vi "信号光谱9 - BN_5.10.vi"() -> ()   [LabVIEW 2018]
uses:
  <vilib>/Utility/NIReport.llb/Report Type.ctl
  <vilib>/Utility/file.llb/Write Delimited Spreadsheet (DBL).vi
  <vilib>/Instr/_visa.llb/VISA Configure Serial Port (Instr).vi
  <vilib>/addons/_office/excel.llb/Excel Get Data ([str]).vi
  <vilib>/Utility/NIReport.llb/NI_report.lvclass
  <vilib>/Analysis/NI_AALBase.lvlib
  <vilib>/ptbypt/NI_PtbyPt.lvlib
  <vilib>/Utility/NIReport.llb/NI_ReportGenerationCore.lvlib
  <vilib>/addons/_office/NI_ReportGenerationToolkit.lvlib
  <vilib>/Utility/NIReport.llb/Excel/NI_Excel.lvclass
panel:
  out "error out 2":errorcluster caption="错误输出"
  out "错误输出":errorcluster
  in  "超时毫秒(25000)":i32=20000
  in  "读取的字节":i32=7
  in  "格式字符串":string
  in  "分隔符(Tab)":string=","
  in  "端口":u16=65432
  in  "地址":string="127.0.0.1"
  out "原始峰值":dbl
  out "拟合峰值":dbl
  in  "角度倍乘系数":dbl=1.5
  out "结果展示":dbl[][](array[numeric])=[[37.33100777239877, 2672.955043835526, 29.54153292599307, 222755.0, 50.0], [37.36593979472361, 2672.656498058864, 30.113284142729572, 222833.0, 50.0], [38.96986225690859, 2673.3337152325566, 33.38805102415213, 222910.0, 75.0], [37.39946104045098, 2676.4005085744548, 31.215565446104666, 222948.0, 47.0], [35.862209164247574, 2671.7826876859012, 30.355582265151796, 223028.0, 47.0]]
  out "Δw2>C":bool=TRUE
  out "Δw1>C":bool=TRUE
  out "θi":dbl
  in  "w0":dbl format="%#_13g"
  in  "C=w-w0":dbl=180.0 format="%#_13g"
  in  "上升下降沿/s":dbl format="%.2p"
  in  "延时/s":dbl format="%.2p"
  in  "占空比/%":dbl=3.0 format="%.2p"
  in  "高电平/V":dbl=4.0 format="%.2p"
  in  "频率/Hz":dbl=6000.0 format="%.3p"
  in  "低电平/V":dbl min=0.0 max=5.0 format="%.2p"
  in  "Enable":bool
  in  "上升下降沿":i32(ring)=1 items=["上升沿", "下降沿"]
  in  "输出信号波形":u16(ring) items=["Pulse"]
  out "Output":bool
  in  "VISA 信号发生器":refnum<visa-resource-name>="USB0::0x1AB1::0x0641::DG4E192200870::INSTR"
  out "Output 2":bool
  in  "Enable 2":bool
  in  "上升下降沿/s 2":dbl format="%.2p"
  in  "延时/s 2":dbl format="%.2p"
  in  "占空比/% 2":dbl=3.0 format="%.2p"
  in  "高电平/V 2":dbl=0.002 format="%.2p"
  in  "频率/Hz 2":dbl=6000.0 format="%.3p"
  in  "低电平/V 2":dbl min=0.0 max=5.0 format="%.2p"
  in  "上升下降沿 2":i32(ring)=1 items=["上升沿", "下降沿"]
  in  "输出信号波形 2":u16(ring) items=["Pulse"]
  in  "终止测量":bool
  in  "测量次数":i32=1
  out "best fit":cluster{"Y":dbl[], "Y":dbl[]}[](graph)
  in  "拟合终点":i32=850
  in  "拟合起点":i32=200
  out "angle":dbl
  out "图片地址":string
  in  "开光时间/ms":u32=50
  out "最终存储路径 2":path
  out "照明光error out":errorcluster
  in  "照明光":bool
  in  "stop bits (10: 1 bit)":u16(ring)=10 items=["1.0"=10, "1.5"=15, "2.0"=20]
  in  "parity (0:none)":enum16{"None", "Odd", "Even", "Mark", "Space"}(ring)
  in  "data bits (8)":u16=8 min=5 max=8 step=1
  in  "baud rate":u32=9600 caption="baud rate (115200)" min=9600 max=115200
  in  "照明光VISA":refnum<visa-resource-name>="COM13"
  out "正在测量":bool
  in  "滤波阈值":dbl=3000.0 format="%#_13g"
  out "范围内？":bool[](array[boolean])
  out "w":dbl
  out "xc":dbl
  out "拟合参数":dbl[](array[numeric])
  out "最终存储路径":path
  in  "停止程序":bool
  out "configure error out":errorcluster
  in  "设置参数":bool
  out "output control error  4":errorcluster
  in  "低电平持续输出":bool
  out "output control error  5":errorcluster
  out "output control error":errorcluster
  in  "开始测量":bool
  in  "channel输出口":i32(ring) items=["Channel 1", "Channel 2"]
  out "output control error":errorcluster
  out "Spectrum":cluster{"Y":dbl[], "Y":dbl[]}[](graph)
  out "波长范围":dbl[](array[numeric])
  in  "?":enum32{"IHR 550", "CCD"}(tab)
  in  "Move To\nTarget Positions":bool
  out "Current UniqueID":string="Mono4"
  in  "Mono ID":string(combo)="Mono1"
  in  "Connect":bool
  out "Initialized JY":bool=TRUE
  in  "Force\nInitialization":bool
  in  "Target Grating":string(combo)="2"
  out "Current Description":string="1" caption="Description"
  out "Grating Index":i32=1
  out "Current Grating":dbl=1200.0
  out "Units":string="nm"
  out "Current WL":dbl=897.9988
  out "Exit Mirror\nPosition":i32(ring)=2 items=["EntranceMirror", "ExitMirror", "Front", "Side"]
  out "Entrance Mirror\nPosition":i32(ring)=2 items=["EntranceMirror", "ExitMirror", "Front", "Side"]
  out "Units 2":string="mm"
  out "Front Entrance":dbl
  in  "Target WL":dbl=516.0
  in  "Exit Mirror":u16(ring)=3 caption="Target Position Exit Mirror" items=["Front"=2, "Side"=3]
  in  "Entrance Mirror":u16(ring)=2 caption="Target Position\nEntrance Mirror" items=["Front"=2, "Side"=3]
  in  "Target\nFront Entrance":dbl=2.0
  in  "Commande tab":T1(tab)
  in  "Area Number to Display":i32
  in  "Reformat":bool
  in  "GAIN":u16(ring)=2 caption="Device Name" items=["High Light", "Best Dynamic Range", "High Sensitivity"]
  in  "ADC":u16(ring) caption="Device Name" items=["20 kHz       ", " 1 MHz       ", " 1 MHz Ultra "]
  in  "Number of Areas :":u16=1 min=1 step=1
  in  "Integration time (ms) :":i16=20000
  out "Uniques ID":u16(ring) items=["CCD1", "CCD2"]
  in  "Device Name":u16(ring) items=["Synapse CCD (Lateral)", "Synapse_IGA (Axial)"]
  in  "Signal type :":enum16{"TTL Rising Edge", "TTL Falling Edge"}(ring)=enum."TTL Falling Edge"
  in  "Trigger Type :":u16(ring) items=["On Start"=1, "Per Acquisition"=2]
  in  "trigSigTypeString":string
  in  "trigEventString":string
  in  "Enable InputTriggers :":bool
  in  "Number of Cleans":i32=1
  in  "MultiAcqShutterMode":i32(ring)=3 items=["Open For All Spectra"=1, "Open for Each Spectrum"=3]
  in  "Accumulations:":u16=10 min=1 step=1
  in  "Multi Accumulation mode:":bool
  out "Y Pixels:":i32=256
  out "DataSize":i32=1024
  out "X Pixels:":i32=1024
  out "Firmware\nVersion":string="V1.20 CCD_4000"
  out "initialized ?":bool=TRUE
  in  "Continuous":bool
  in  "CCD Busy":bool
  out "indicator":string="Ready !"
  in  "initialize":bool
  in  "ShutterOpen":bool=TRUE caption="Shutter enable"
  in  "Acquire":bool
  in  "Temperature":bool
  in  "Setup":bool
  out "Acq Time(ms)":u32=3401
  in  "Save Backlight":bool
  in  "cut backlight":bool
  out "backlight":bool=TRUE
  in  "是否拟合":bool
  in  "是否保存":bool
  in  "Close":bool=TRUE
  out "JYCCDLib.IJYCCDReqd":refnum<k7>
  out "areas :":i32[][](array[numeric])=[[1], [1], [1], [1024], [256], [1], [256]]
  in  "Constante de condition\n(Voir l'aide contextuelle)":bool
  out "temp graph":dbl(graph)=-134.538067
  out "ADC Number":i32[](array[numeric])=[0, 1, 2, 3, 4]
  out "Gain Number":i32[](array[numeric])=[10, 11, 12, 13, 8, 2]
  out "trigAddress":i32
  out "Data":i32[][](graph)
  out "error out":errorcluster
  out "Gratings":dbl[](array[numeric])=[1200.0, 300.0]
  out "Backlight":i32[][](graph)
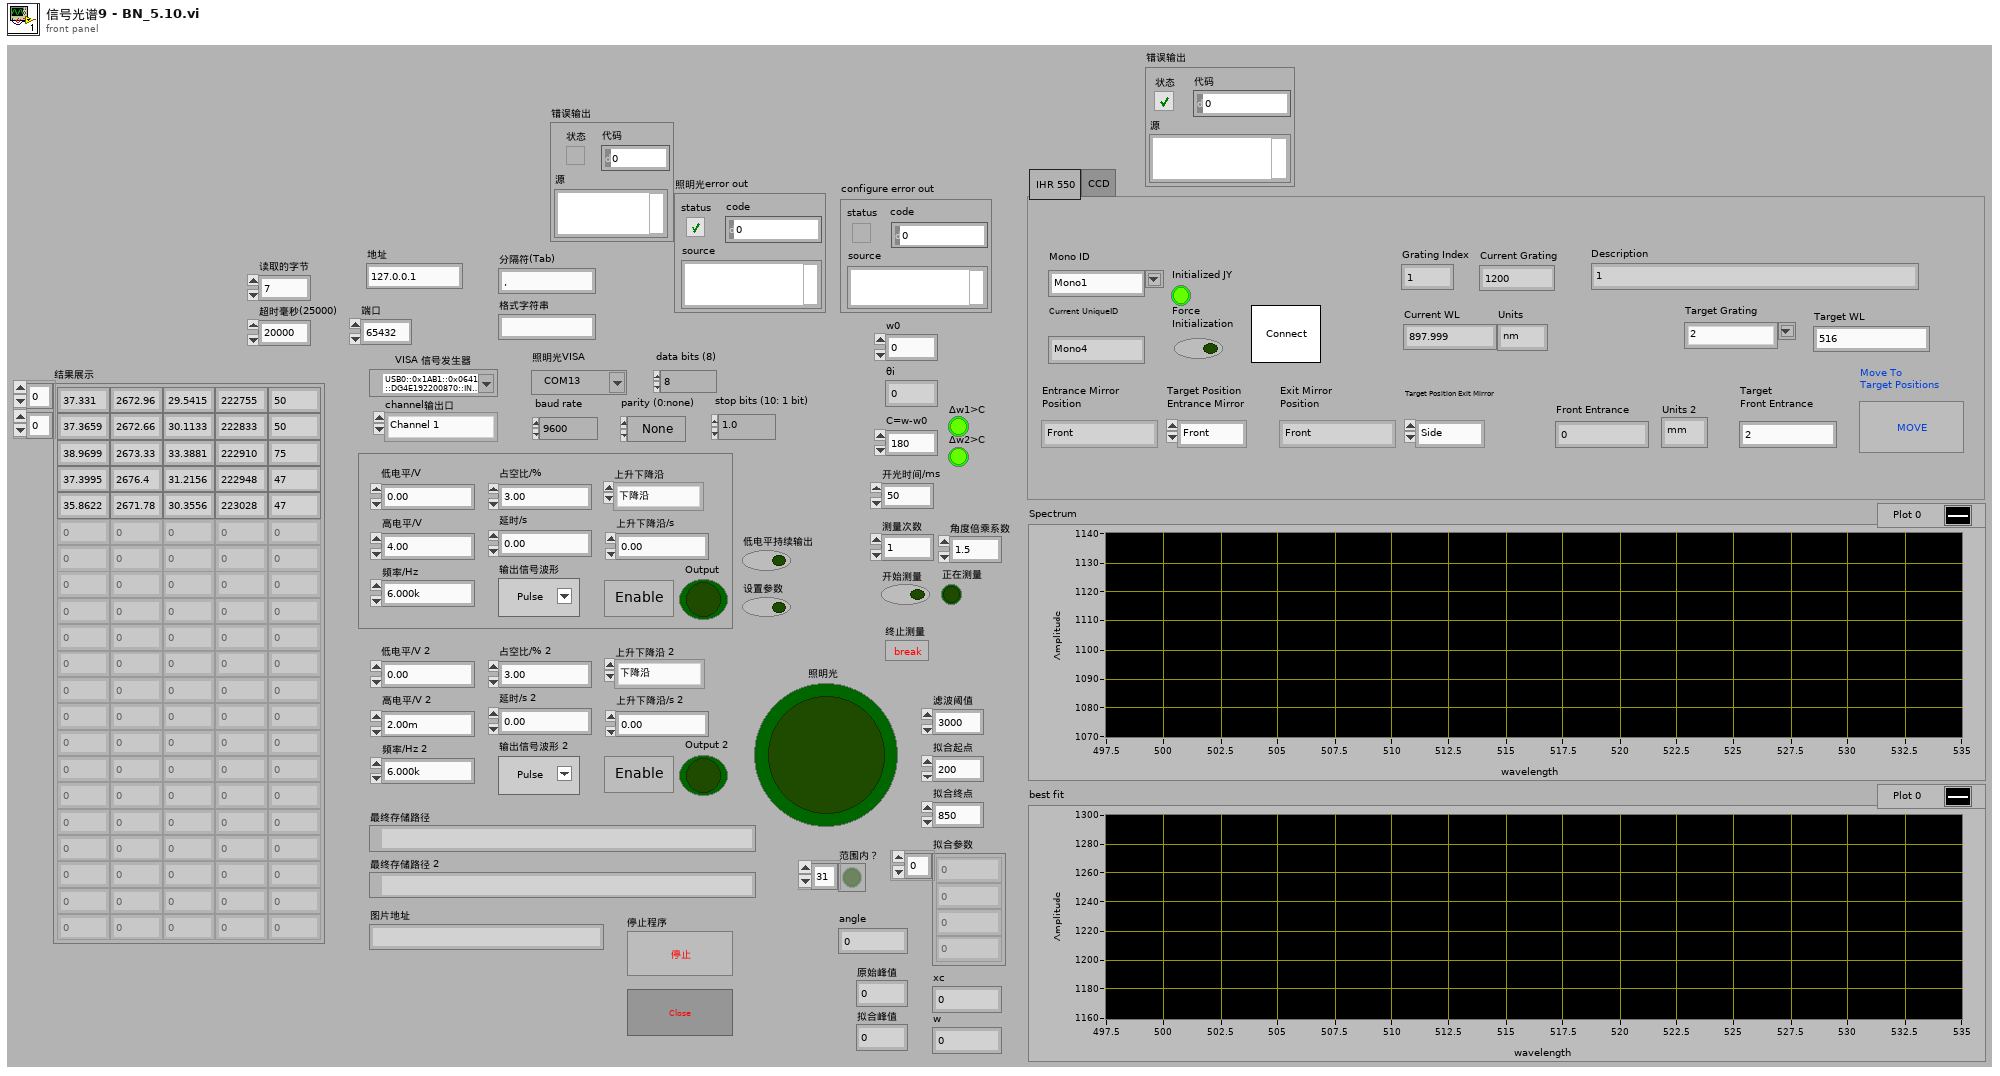
[diagram p1: front panel]
types:
  T1 = enum32{"Settings", "Trigger In", "Multi-Accu.", "Infos"}
  T2 = enum8{"Enabled", "Disabled", "Disabled and Grayed Out"}
  T3 = enum16{"maximized", "minimized", "normal", "no change"}
  T4 = typedef "NI_ReportGenerationCore.lvlib/Report Type.ctl" = enum16{"HTML", "Word", "Excel"}
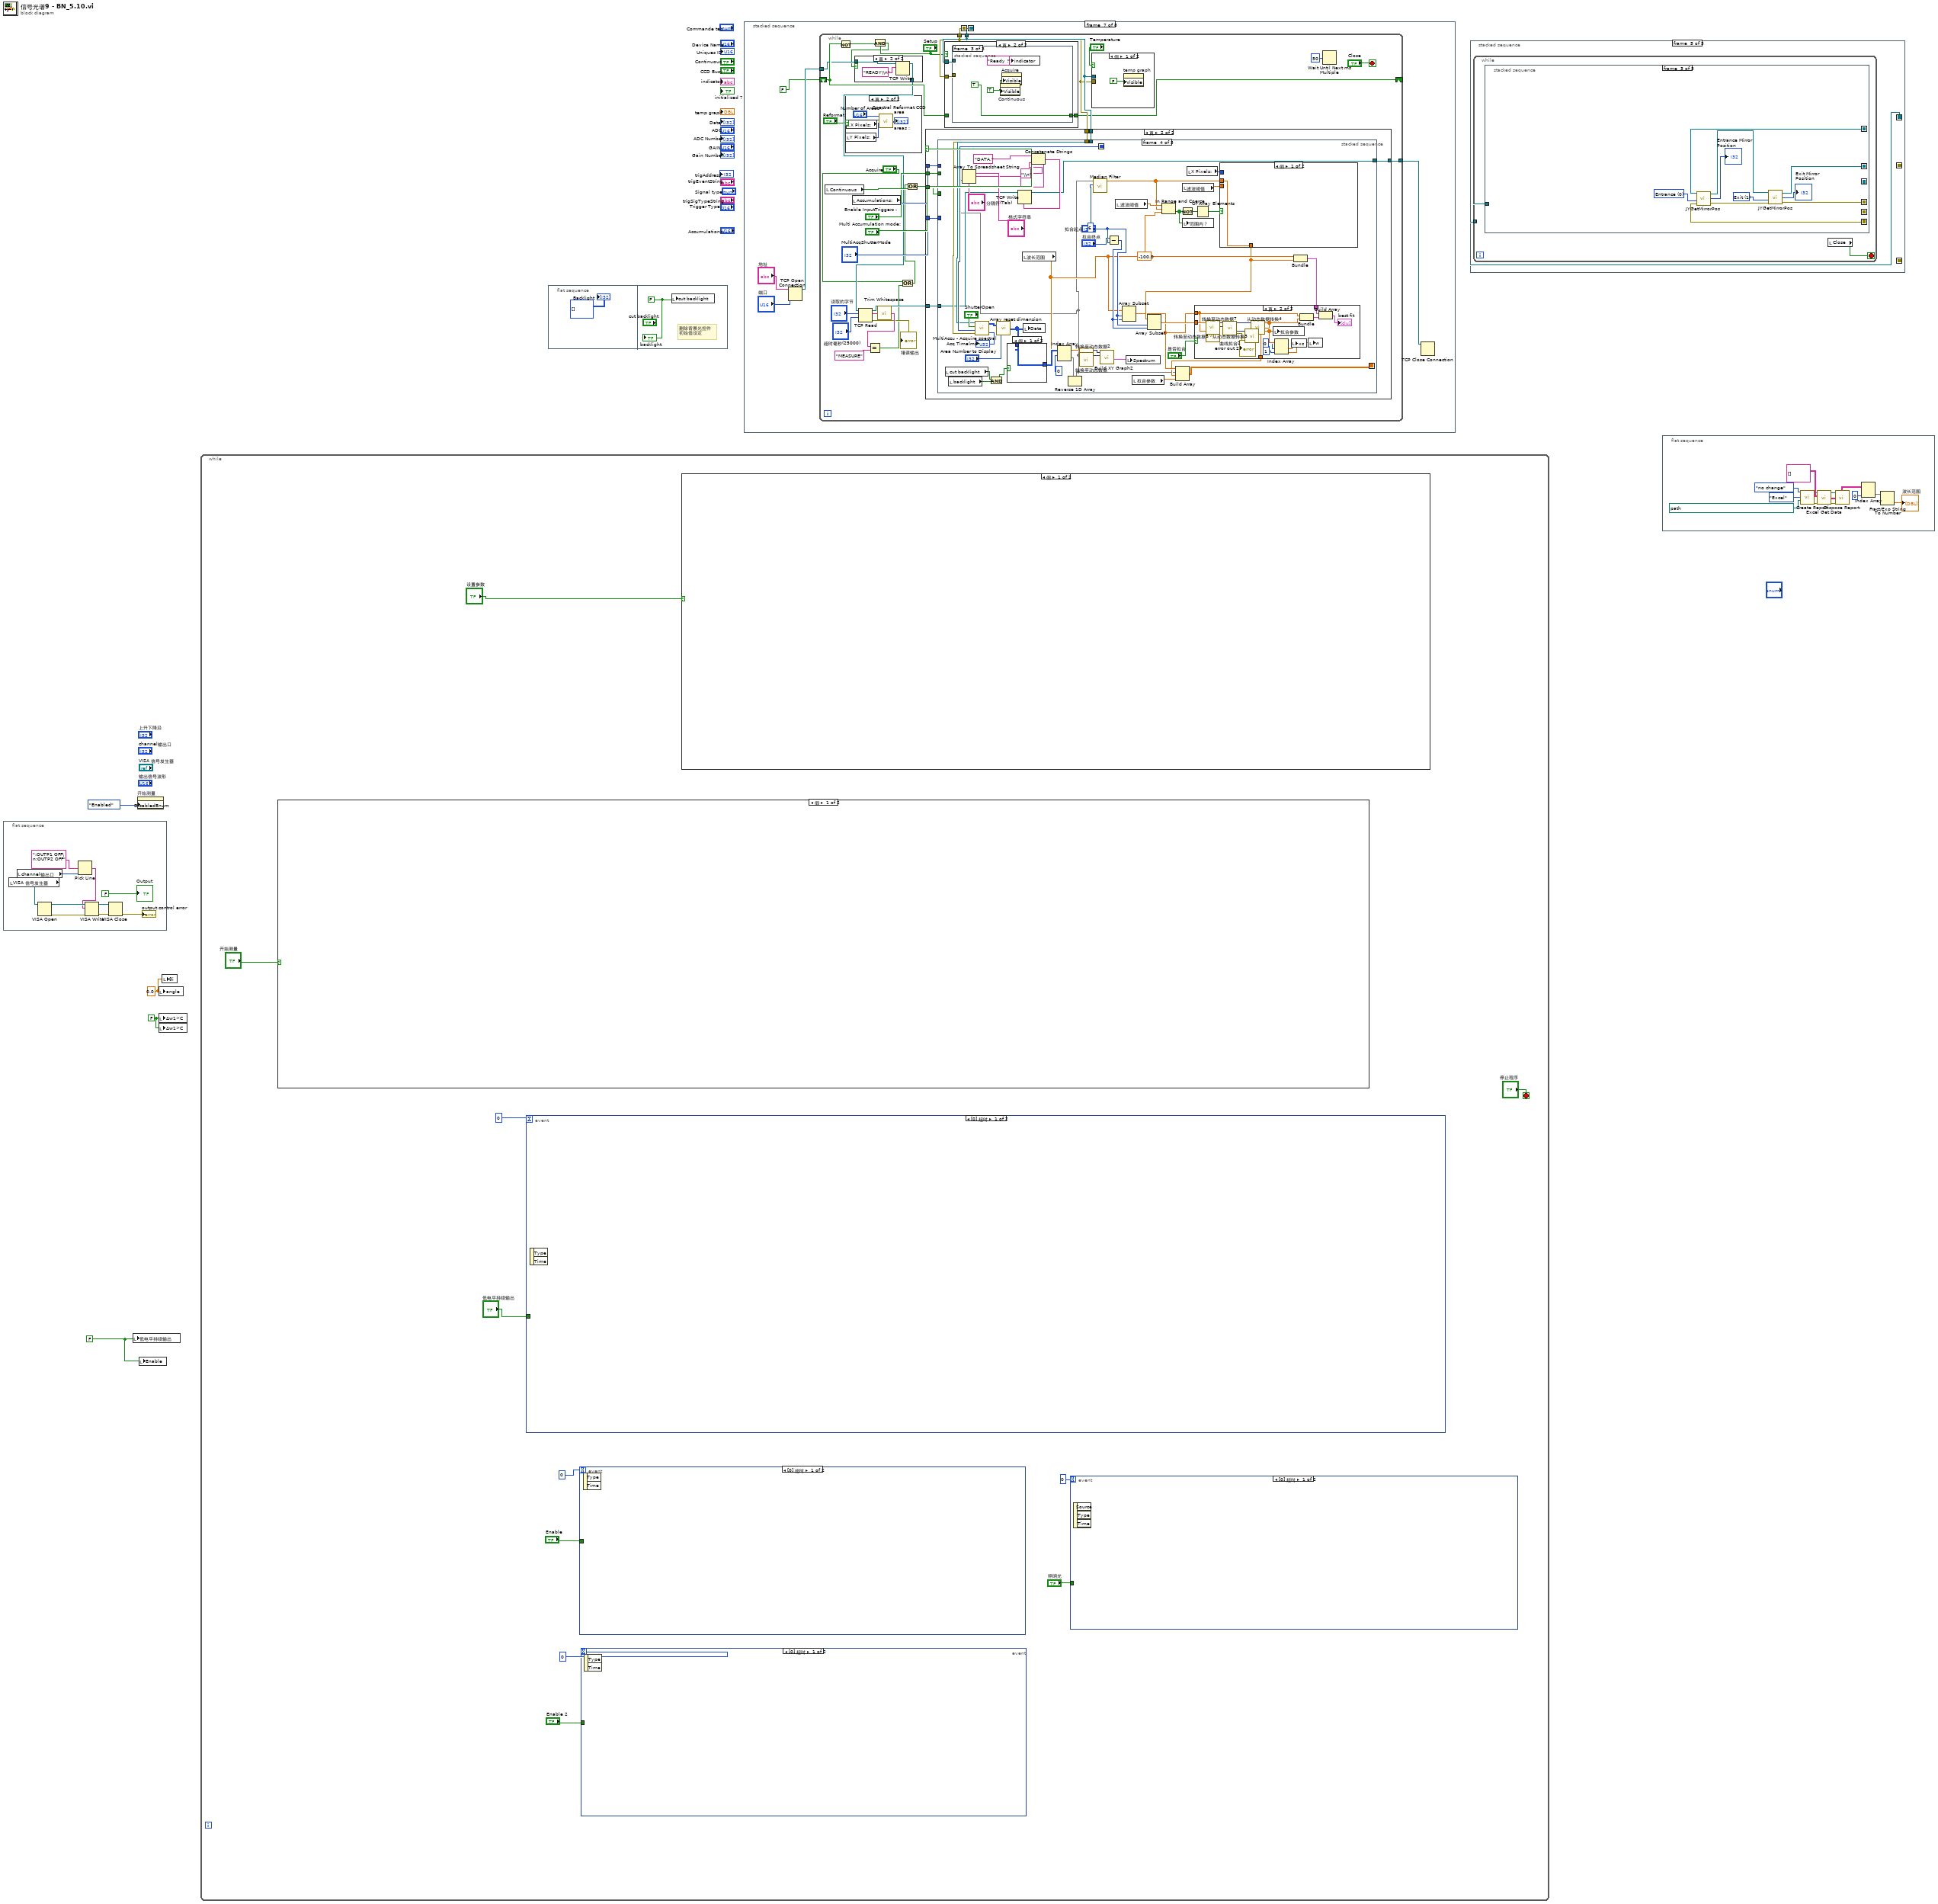
[diagram p0: block diagram]
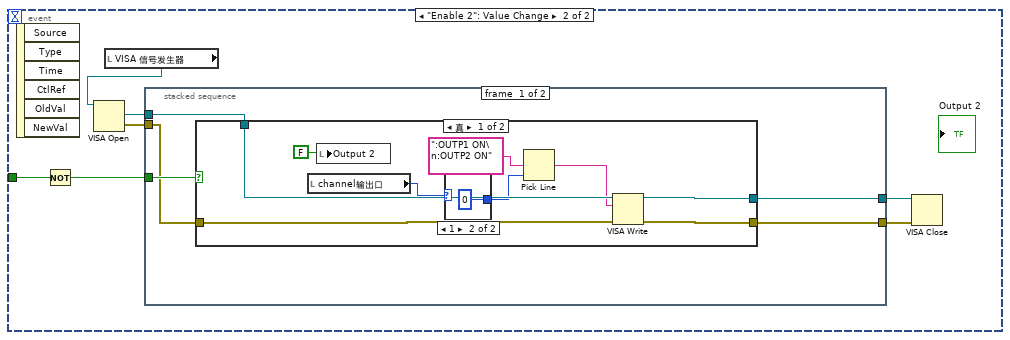
[diagram p2: hidden frame]
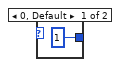
[diagram p3: hidden frame]
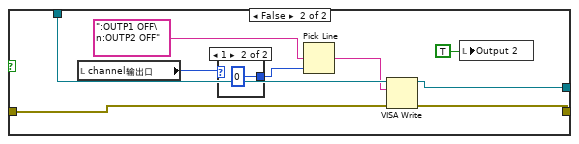
[diagram p4: hidden frame]
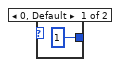
[diagram p5: hidden frame]
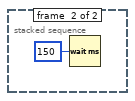
[diagram p6: hidden frame]
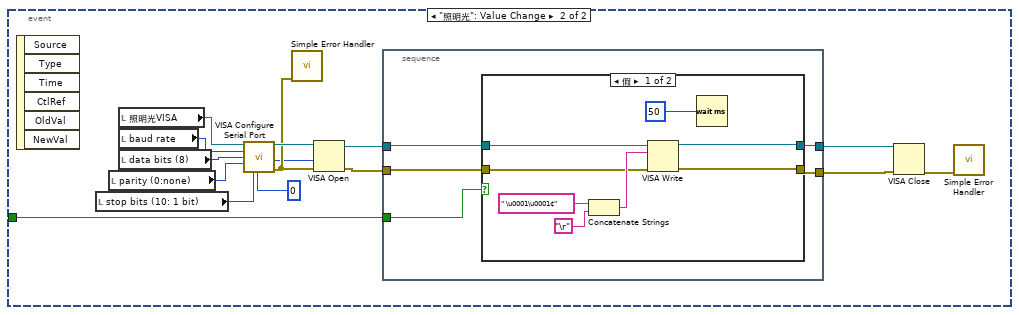
[diagram p7: hidden frame]
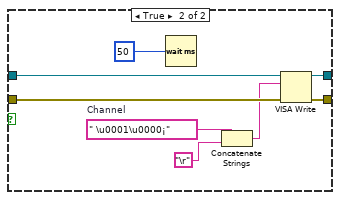
[diagram p8: hidden frame]
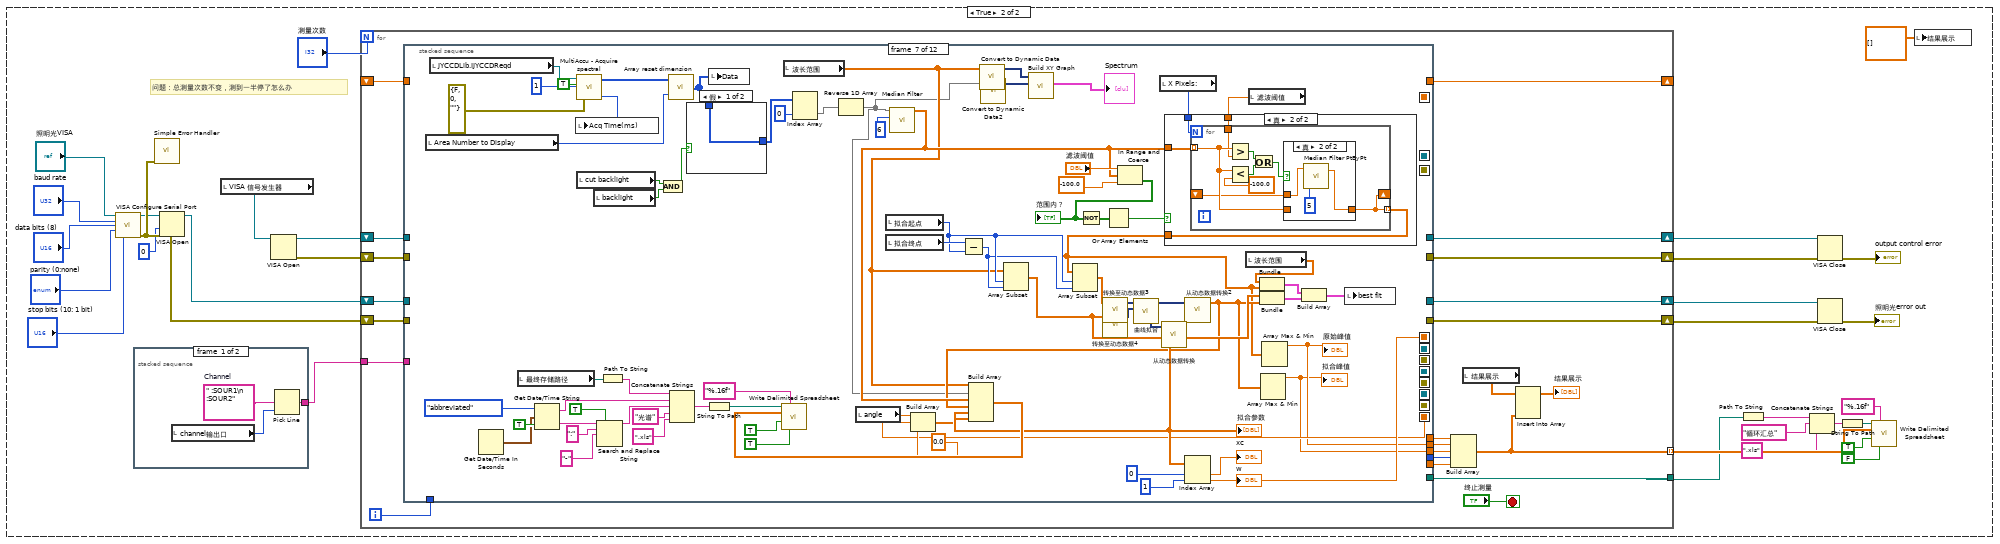
[diagram p9: hidden frame]
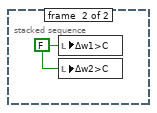
[diagram p10: hidden frame]
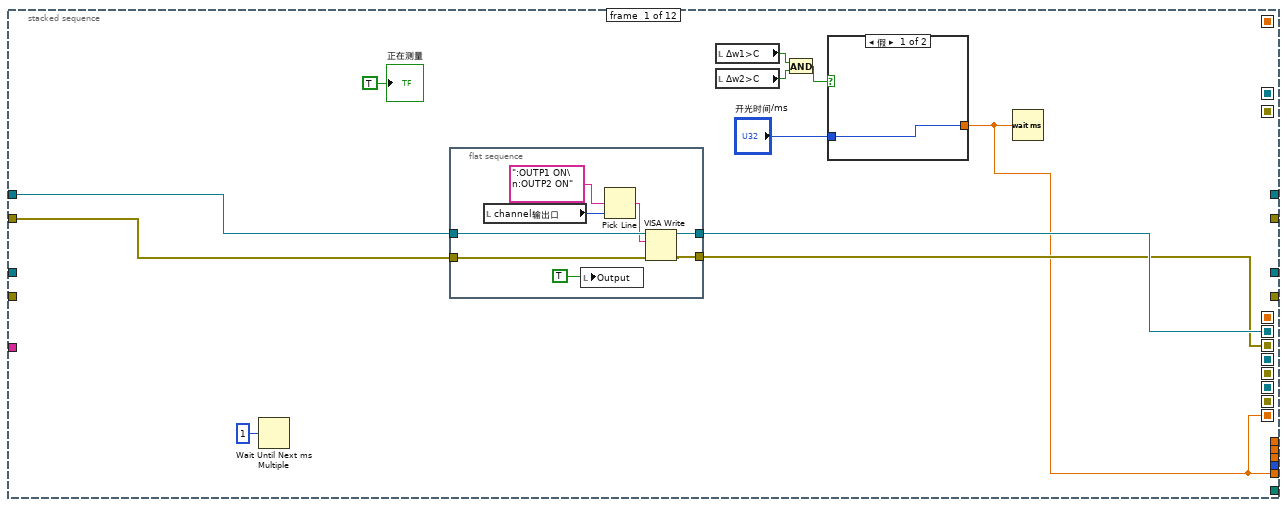
[diagram p11: hidden frame]
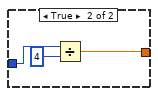
[diagram p12: hidden frame]
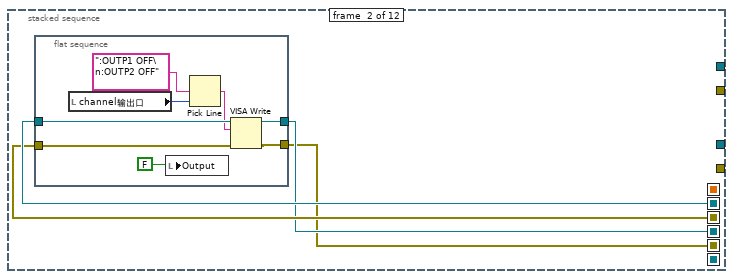
[diagram p13: hidden frame]
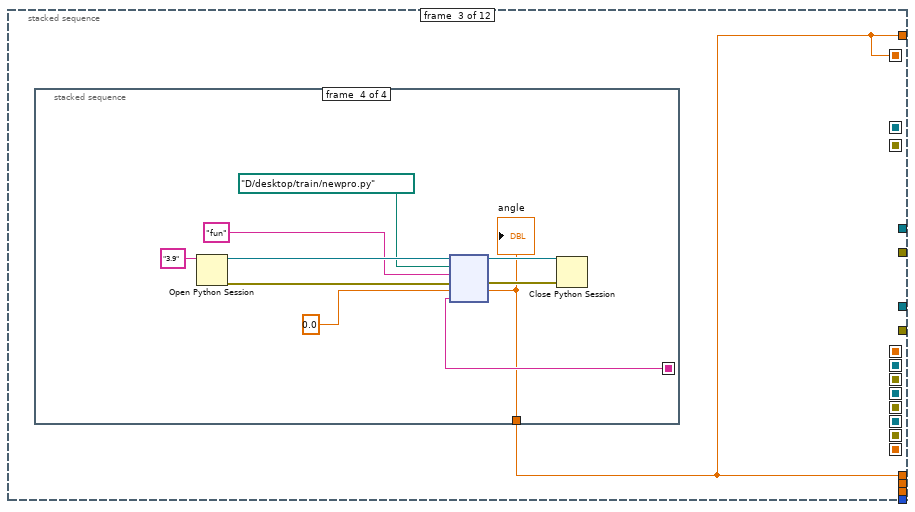
[diagram p14: hidden frame]
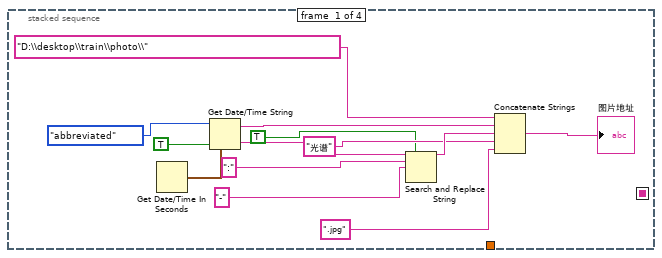
[diagram p15: hidden frame]
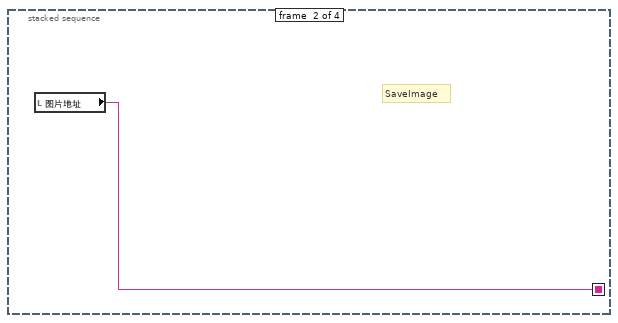
[diagram p16: hidden frame]
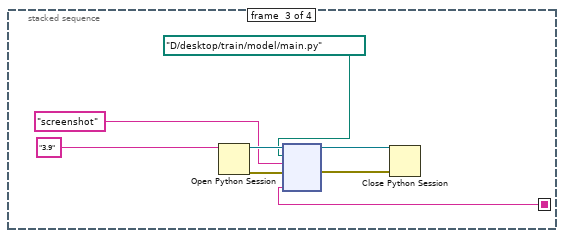
[diagram p17: hidden frame]
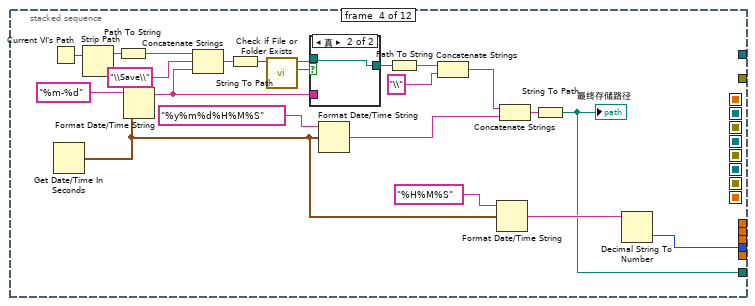
[diagram p18: hidden frame]
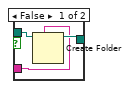
[diagram p19: hidden frame]
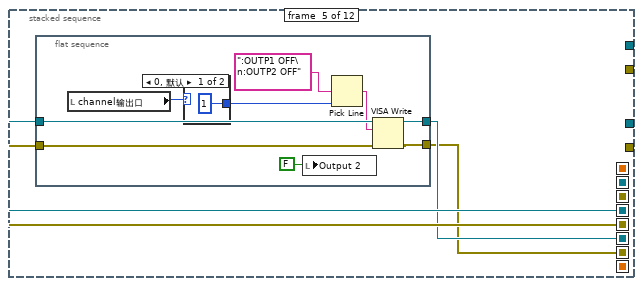
[diagram p20: hidden frame]
diagram:
  w1 = FALSE ("Δw1>C")
  w2 = 0.0 ("angle")
  w3 = FALSE
  n1 = flat-sequence {
    frame #0 {
      n2 = local read "VISA 信号发生器"() -> (w8:refnum<visa-resource-name>)
      n3 = local read "channel输出口"() -> (w6:i32)
      n4 = VISA Open(VISA resource name=w8) -> (VISA resource name=w14:refnum<visa-resource-name>, error out=w13:errorcluster)  [unwired: 4 in]
      n5 = Pick Line(multi-line string=":OUTP1 OFF\n:OUTP2 OFF" ("write buffer"), line index=w6) -> (output string=w5:string)  [unwired: 1 in]
      n6 = VISA Write(VISA resource name=w14, write buffer=w5, error in (no error)=w13) -> (VISA resource name out=w11:refnum<visa-resource-name>, error out=w10:errorcluster)  [unwired: 1 out]
      n7 = VISA Close(VISA resource name=w11, error in (no error)=w10) -> (error out=→"output control error":errorcluster)
      "Output" <- FALSE ("布尔")
    }
  }
  n8 = local write "低电平持续输出"(w3) -> ()
  n9 = property on="开始测量" class="Bool"("DisabledEnum"=T2."Enabled" ("禁用")) -> ()  [unwired: 2 in, 2 out]
  n10 = local write "Enable"(w3) -> ()
  n11 = local write "angle"(w2) -> ()
  n12 = local write "Δw1>C"(w1) -> ()
  n13 = local write "Δw1>C"(w1) -> ()
  n14 = local write "θi"(w2) -> ()
  n15 = while {
    stop <- "停止程序" stop-if-true
    n16 = case shown="假" "开始测量" {
      frame False {
      }
      frame True {
        # "问题：总测量次数不变，测到一半停了怎么办"
        n17 = call-poly "VISA Configure Serial Port"("VISA resource name"="照明光VISA", "baud rate (9600)"="baud rate", "data bits (8)"="data bits (8)", "parity (0:none)"="parity (0:none)", "stop bits (10: 1 bit)"="stop bits (10: 1 bit)") -> ("VISA resource name out"=w118:refnum<visa-resource-name>, "error out"=w119:errorcluster)  [unwired: 9 in]
        n18 = stacked-sequence {
          tunnel: [w128 _] -> w122
          frame #0 {
            w129 = " :SOUR1\n :SOUR2"  # Channel
            n19 = local read "channel输出口"() -> (w130:i32)
            n20 = Pick Line(multi-line string=w129, line index=w130) -> (output string=w128:string)  [unwired: 1 in]
          }
          frame #1 {
            w131 = FALSE ("Δw1>C")
            n21 = local write "Δw1>C"(w131) -> ()
            n22 = local write "Δw2>C"(w131) -> ()
          }
        }
        n23 = call <vilib>:"Simple Error Handler.vi"("error in (no error)"=w119) -> ()  [unwired: 4 in, 5 out]
        n24 = VISA Open(access mode=0, error in (no error)=w119, VISA resource name=w118) -> (VISA resource name=w111:refnum<visa-resource-name>, error out=w110:errorcluster)  [unwired: 2 in]
        n25 = local read "VISA 信号发生器"() -> (w127:refnum<visa-resource-name>)
        n26 = VISA Open(VISA resource name=w127) -> (VISA resource name=w126:refnum<visa-resource-name>, error out=w125:errorcluster)  [unwired: 4 in]
        n27 = for {
          N: "测量次数" -> [_]
          tunnel: w122 -> [w151]
          shift-right: [w147] -> w121
          shift-left: w126 -> [w153]
          shift-right: [w146] -> w120
          shift-left: w125 -> [w152]
          shift-right: [w145] -> w124
          shift-left: w111 -> [w150]
          shift-right: [w144] -> w123
          shift-left: w110 -> [w149]
          tunnel: [w134] -> w100 mode=indexing
          shift-right: [w139] -> _
          shift-left: _ -> [w138]
          tunnel: [w135] -> w97
          i -> [w137]
          stop <- "终止测量" stop-if-true
          n28 = stacked-sequence {
            seq-local: [w160 _ _ _ _ _ _ _ _ _ _ _] -> [_ w180 _ _ _ _ _ _ _ _ _ _]
            seq-local: [w159 _ _ _ _ _ _ _ _ _ _ _] -> [_ w179 _ _ _ _ _ _ _ _ _ _]
            seq-local: [_ _ _ _ _ w265 _ _ _ _ _ _] -> [_ _ _ _ _ _ _ _ w383 _ _ _]
            seq-local: [_ _ _ _ _ w264 _ _ _ _ _ _] -> [_ _ _ _ _ _ _ _ w386 _ _ _]
            seq-local: [_ w178 _ _ _ _ _ _ _ _ _ _] -> [_ _ _ _ w251 _ _ _ _ _ _ _]
            seq-local: [_ w177 _ _ _ _ _ _ _ _ _ _] -> [_ _ _ _ w250 _ _ _ _ _ _ _]
            seq-local: [_ _ _ _ w249 _ _ _ _ _ _ _] -> [_ _ _ _ _ _ _ w369 _ _ _ _]
            seq-local: [_ _ _ _ w248 _ _ _ _ _ _ _] -> [_ _ _ _ _ _ _ w368 _ _ _ _]
            seq-local: [_ _ w189 _ _ _ _ _ _ _ _ _] -> [_ _ _ _ _ _ _ _ _ _ w395 _]
            seq-local: [_ _ _ _ _ _ w280 _ _ _ _ _] -> [_ _ _ _ _ _ _ _ _ _ w390 _]
            seq-local: [w154 _ _ _ _ _ _ _ _ _ _ _] -> [_ _ _ _ _ _ w278 _ _ _ _ _]
            tunnel: w153 -> [w162 _ _ _ _ _ _ _ _ _ _ _]
            tunnel: w152 -> [w161 _ _ _ _ _ _ _ _ _ _ _]
            tunnel: [_ _ _ _ _ _ _ w367 _ _ _ _] -> w147
            tunnel: [_ _ _ _ _ _ _ w366 _ _ _ _] -> w146
            tunnel: w151 -> [_ _ _ _ _ _ _ _ _ _ _ _]
            tunnel: w150 -> [_ _ _ _ _ w268 _ _ _ _ _ _]
            tunnel: w149 -> [_ _ _ _ _ w267 _ _ _ _ _ _]
            tunnel: [_ _ _ _ _ _ _ _ w385 _ _ _] -> w145
            tunnel: [_ _ _ _ _ _ _ _ w384 _ _ _] -> w144
            tunnel: [_ _ w189 _ _ _ _ _ _ _ _ _] -> w143
            tunnel: [_ _ _ _ _ _ w275 _ _ _ _ _] -> w142
            tunnel: [_ _ _ _ _ _ w274 _ _ _ _ _] -> w141
            tunnel: [_ _ _ w223 _ _ _ _ _ _ _ _] -> w140
            tunnel: [w154 _ _ _ _ _ _ _ _ _ _ _] -> w136
            tunnel: [_ _ w189 _ _ _ _ _ _ _ _ _] -> w139
            tunnel: w138 -> [_ _ _ _ _ _ _ _ _ _ w394 _]
            tunnel: w137 -> [_ _ _ _ _ _ _ _ _ _ w392 _]
            tunnel: [_ _ _ w222 _ _ _ _ _ _ _ _] -> w135
            frame #0 {
              n29 = Wait Until Next ms Multiple(millisecond multiple=u32 1 ("毫秒倍数")) -> ()  [unwired: 1 out]
              n30 = flat-sequence {
                tunnel: w162 -> [w176]
                tunnel: w161 -> [w175]
                tunnel: [w170] -> w160
                tunnel: [w169] -> w159
                frame #0 {
                  n31 = local read "channel输出口"() -> (w172:i32)
                  n32 = local write "Output"(TRUE ("布尔")) -> ()
                  n33 = Pick Line(multi-line string=":OUTP1 ON\n:OUTP2 ON" ("write buffer"), line index=w172) -> (output string=w171:string)  [unwired: 1 in]
                  n34 = VISA Write(VISA resource name=w176, write buffer=w171, error in (no error)=w175) -> (VISA resource name out=w170:refnum<visa-resource-name>, error out=w169:errorcluster)  [unwired: 1 out]
                }
              }
              n35 = local read "Δw1>C"() -> (w156:bool)
              n36 = local read "Δw2>C"() -> (w157:bool)
              n37 = And(x=w156, y=w157) -> (x .and. y?=w155:bool)
              n38 = case shown="假" w155 {
                tunnel: [w165 w166] -> w154
                tunnel: "开光时间/ms" -> [w165 w168]
                frame False {
                }
                frame True {
                  n39 = Divide(x=w168, y=u32 4) -> (x/y=w166:dbl)
                }
              }
              n40 = Wait (ms)(milliseconds to wait=w154) -> ()  [unwired: 1 out]
              "正在测量" <- TRUE
            }
            frame #1 {
              n41 = flat-sequence {
                tunnel: w180 -> [w188]
                tunnel: w179 -> [w187]
                tunnel: [w182] -> w178
                tunnel: [w181] -> w177
                frame #0 {
                  n42 = local read "channel输出口"() -> (w184:i32)
                  n43 = local write "Output"(FALSE ("布尔")) -> ()
                  n44 = Pick Line(multi-line string=":OUTP1 OFF\n:OUTP2 OFF" ("write buffer"), line index=w184) -> (output string=w183:string)  [unwired: 1 in]
                  n45 = VISA Write(VISA resource name=w188, write buffer=w183, error in (no error)=w187) -> (VISA resource name out=w182:refnum<visa-resource-name>, error out=w181:errorcluster)  [unwired: 1 out]
                }
              }
            }
            frame #2 {
              n46 = stacked-sequence {
                seq-local: [_ w203 _ _] -> [_ _ w204 w213]
                tunnel: [_ _ _ w212] -> w189
                frame #0 {
                  n47 = Get Date/Time In Seconds() -> (seconds since 1Jan1904=w199:timestamp)
                  n48 = Get Date/Time String(date format (0)=enum16{"short", "long", "abbreviated"}."abbreviated" ("日期格式(0)"), seconds (now)=w199, want seconds? (F)=TRUE ("需要秒？(F)")) -> (date string=w202:string, time string=w200:string)
                  n49 = Search and Replace String(replace all?=TRUE ("替换全部？(F)"), input string=w200, search string=":" ("搜索字符串"), replace string="-" ("替换字符串(\"\")")) -> (result string=w201:string)  [unwired: 4 in, 3 out]
                  n50 = Concatenate Strings("D:\\desktop\\train\\photo\\", w202, w201, "光谱" ("字符串"), ".jpg" ("字符串")) -> (→"图片地址":string)
                }
                frame #1 {
                  # "SaveImage"
                  n51 = local read "图片地址"() -> (w203:string)
                }
                frame #2 {
                  n52 = Open Python Session(python version="3.9" ("Python version")) -> (session out=w211:refnum<k35>, error out=w209:errorcluster)  [unwired: 2 in]
                  n53 = node(w211, path "D:/desktop/train/model/main.py" ("module path"), "screenshot" ("function name"), w209, w204) -> (w210:refnum<k35>, w208:errorcluster)  [unwired: 3 in, 2 out]
                  n54 = Close Python Session(session in=w210, error in=w208) -> ()  [unwired: 1 out]
                }
                frame #3 {
                  n55 = Open Python Session(python version="3.9" ("Python version")) -> (session out=w220:refnum<k35>, error out=w218:errorcluster)  [unwired: 2 in]
                  n56 = node(w220, path "D:/desktop/train/newpro.py" ("module path"), "fun" ("function name"), w218, 0.0, w213) -> (w219:refnum<k35>, w217:errorcluster, w212:dbl)  [unwired: 1 in, 2 out]
                  "angle" <- w212
                  n57 = Close Python Session(session in=w219, error in=w217) -> ()  [unwired: 1 out]
                }
              }
            }
            frame #3 {
              n58 = Current VI's Path() -> (path=w232:path)
              n59 = Get Date/Time In Seconds() -> (seconds since 1Jan1904=w225:timestamp)
              n60 = Strip Path(path=w232) -> (stripped path=w233:path)  [unwired: 1 out]
              n61 = Path To String(path=w233) -> (string=w234:string)
              n62 = Format Date/Time String(time format string (%c)="%m-%d" ("时间格式字符串(%c)"), seconds (now)=w225) -> (date/time string=w240:string)  [unwired: 1 in]
              n63 = Concatenate Strings(w234, "\\Save\\" ("字符串"), w240) -> (w235:string)
              n64 = String To Path(string=w235) -> (path=w236:path)
              n65 = call <vilib>:"Check if File or Folder Exists.vi"("path"=w236) -> ("file or folder exists?"=w237:bool, "dup path"=w239:path)  [unwired: 8 in, 1 out]
              n66 = case shown="真" w237 {
                tunnel: [w246 w247] -> w238
                tunnel: w239 -> [w245 w247]
                tunnel: w240 -> [w244 _]
                frame False {
                  n67 = Create Folder(prompt (Create Folder)=w244, path (use dialog)=w245) -> (created path=w246:path)  [unwired: 1 in, 2 out]
                }
                frame True {
                }
              }
              n68 = Format Date/Time String(time format string (%c)="%y%m%d%H%M%S" ("时间格式字符串(%c)"), seconds (now)=w225) -> (date/time string=w243:string)  [unwired: 1 in]
              n69 = Path To String(path=w238) -> (string=w241:string)
              n70 = Concatenate Strings(w241, "\\" ("字符串")) -> (w242:string)
              n71 = Format Date/Time String(time format string (%c)="%H%M%S" ("时间格式字符串(%c)"), seconds (now)=w225) -> (date/time string=w224:string)  [unwired: 1 in]
              n72 = Concatenate Strings(w242, w243) -> (w231:string)
              n73 = String To Path(string=w231) -> (path=w222:path)
              "最终存储路径" <- w222
              n74 = Decimal String To Number(string=w224) -> (number=w223:i32)  [unwired: 2 in, 1 out]
            }
            frame #4 {
              n75 = flat-sequence {
                tunnel: w251 -> [w260]
                tunnel: w250 -> [w259]
                tunnel: [w255] -> w249
                tunnel: [w254] -> w248
                frame #0 {
                  n76 = local read "channel输出口"() -> (w253:i32)
                  n77 = case shown="0, 默认" w253 {
                    tunnel: [1 0] -> w252
                    frame 0, Default {
                    }
                    frame 1 {
                    }
                  }
                  n78 = local write "Output 2"(FALSE ("布尔")) -> ()
                  n79 = Pick Line(multi-line string=":OUTP1 OFF\n:OUTP2 OFF" ("write buffer"), line index=w252) -> (output string=w256:string)  [unwired: 1 in]
                  n80 = VISA Write(VISA resource name=w260, write buffer=w256, error in (no error)=w259) -> (VISA resource name out=w255:refnum<visa-resource-name>, error out=w254:errorcluster)  [unwired: 1 out]
                }
              }
            }
            frame #5 {
              w263 = " \u0001\u0001¢"  # Channel
              n81 = Wait (ms)(milliseconds to wait=1200) -> ()  [unwired: 1 out]
              n82 = Concatenate Strings(w263, "\r") -> (w269:string)
              n83 = local write "照明光"(FALSE ("照明光")) -> ()
              n84 = VISA Write(VISA resource name=w268, write buffer=w269, error in (no error)=w267) -> (VISA resource name out=w265:refnum<visa-resource-name>, error out=w264:errorcluster)  [unwired: 1 out]
            }
            frame #6 {
              n85 = local read "Area Number to Display"() -> (w319:i32)
              n86 = local read "JYCCDLib.IJYCCDReqd"() -> (w315:refnum<k7>)
              n87 = Get Date/Time In Seconds() -> (seconds since 1Jan1904=w328:timestamp)
              n88 = local read "最终存储路径"() -> (w342:path)
              n89 = Get Date/Time String(date format (0)=enum16{"short", "long", "abbreviated"}."abbreviated" ("日期格式(0)"), seconds (now)=w328, want seconds? (F)=TRUE ("需要秒？(F)")) -> (date string=w336:string, time string=w331:string)
              n90 = call "MultiAccu - Acquire spectral.vi"("error in"=errorcluster {"status"=FALSE, "code"=0, "source"=""}, "Accumulations:"=u16 1, "ShutterOpen"=TRUE, "JYCCDLib.IJYCCDReqd"=w315) -> ("Acq Time(ms)"=w321:u32, "Array Out"=w320:i32[][][])  [unwired: 1 out]
              n91 = local write "Acq Time(ms)"(w321) -> ()
              n92 = local read "cut backlight"() -> (w303:bool)
              n93 = local read "backlight"() -> (w301:bool)
              n94 = Search and Replace String(replace all?=TRUE ("替换全部？(F)"), input string=w331, search string=":" ("搜索字符串"), replace string="-" ("替换字符串(\"\")")) -> (result string=w335:string)  [unwired: 4 in, 3 out]
              n95 = Path To String(path=w342) -> (string=w325:string)
              n96 = And(x=w303, y=w301) -> (x .and. y?=w302:bool)
              n97 = call "Array reset dimension.vi"("Area Number"=w319, "Array In"=w320) -> ("Array Out"=w305:i32[][])
              n98 = Concatenate Strings(w325, w336, w335, "光谱" ("字符串"), ".xls" ("字符串")) -> (w340:string)
              n99 = case shown="假" w302 {
                tunnel: [w362 w364] -> w304
                tunnel: w305 -> [w362 w363]
                frame False {
                }
                frame True {
                  n100 = local read "Backlight"() -> (w365:i32[][])
                  n101 = Subtract(x=w363, y=w365) -> (x-y=w364:i32[][])
                }
              }
              n102 = String To Path(string=w340) -> (path=w341:path)
              n103 = local write "Data"(w305) -> ()
              n104 = local read "波长范围"() -> (w273:dbl[])
              n105 = Index Array(array=w304, index (row)=0 ("索引 (行)")) -> (element=w343:i32[])  [unwired: 1 in]
              n106 = Reverse 1D Array(array=w343) -> (reversed array=w272:i32[])
              n107 = local read "angle"() -> (w284:dbl)
              n108 = local read "拟合起点"() -> (w291:i32)
              n109 = local read "拟合终点"() -> (w293:i32)
              n110 = call <vilib>:"Median Filter.vi"("left rank"=6, "X"=w272) -> ("Filtered X"=w282:dbl[])  [unwired: 8 in, 1 out]
              n111 = Build Array(w284, w278, 0.0 ("元素")) -> (w283:dbl[])
              n112 = Subtract(x=w293, y=w291) -> (x-y=w290:i32)
              n113 = call "Convert to Dynamic Data"("Array"=w273) -> ("Dynamic Data Type"=w312:dynamicdata)  [unwired: 3 in]
              n114 = call "Convert to Dynamic Data2"("Array"=w272) -> ("Dynamic Data Type"=w311:dynamicdata)  [unwired: 3 in]
              n115 = Array Subset(array=w273, index=w291, length=w290) -> (w289:dbl[])
              n116 = call "Build XY Graph"("Y Input"=w311, "X Input"=w312) -> ("XY Graph"=→"Spectrum":cluster{"Y":dbl[], "Y":dbl[]}[])  [unwired: 8 in, 1 out]
              n117 = call "转换至动态数据4"("Array"=w289) -> ("Dynamic Data Type"=w309:dynamicdata)  [unwired: 3 in]
              n118 = In Range and Coerce(upper limit="滤波阈值", x=w282, lower limit=-100.0) -> (In Range?=w296:bool[])  [unwired: 1 out]
              "范围内？" <- w296
              n119 = Not(x=w296) -> (.not. x?=w295:bool[])
              n120 = Or Array Elements(Boolean array=w295) -> (logical OR=w298:bool)
              n121 = local read "X Pixels:"() -> (w297:i32)
              n122 = local read "波长范围"() -> (w285:dbl[])
              n123 = local read "滤波阈值"() -> (w294:dbl)
              n124 = case shown="真" w298 {
                tunnel: w297 -> [_ w349]
                tunnel: w282 -> [w345 w348]
                tunnel: [w345 w347] -> w276
                tunnel: w294 -> [_ w346]
                frame False {
                }
                frame True {
                  n125 = for {
                    N: w349 -> [_]
                    tunnel: w348 -> [w353] mode=indexing
                    tunnel: [w352] -> w347 mode=indexing
                    shift-right: [w352] -> _
                    shift-left: _ -> [w351]
                    tunnel: w346 -> [w350]
                    n126 = Greater?(x=w353, y=w350) -> (0:w355:bool)
                    n127 = Less?(x=w353, y=-100.0) -> (x < y?=w356:bool)
                    n128 = Or(x=w355, y=w356) -> (x .or. y?=w354:bool)
                    n129 = case shown="真" w354 {
                      tunnel: w353 -> [w358 _]
                      tunnel: [w358 w360] -> w352
                      tunnel: w351 -> [_ w361]
                      frame False {
                      }
                      frame True {
                        n130 = call <vilib>:"Median Filter PtByPt.vi"("rank"=5, "x"=w361) -> ("Filtered x"=w360:dbl)  [unwired: 2 in, 1 out]
                      }
                    }
                  }
                }
              }
              n131 = Array Subset(array=w276, index=w291, length=w290) -> (w292:dbl[])
              n132 = call "转换至动态数据3"("Array"=w292) -> ("Dynamic Data Type"=w310:dynamicdata)  [unwired: 3 in]
              n133 = call "曲线拟合"("Locations"=w309, "Signals"=w310) -> ("best fit"=w314:dynamicdata, "non-linear coefficients"=w313:dynamicdata)  [unwired: 5 in, 3 out]
              n134 = call "从动态数据转换"("Dynamic Data Type"=w313) -> ("Array"=w306:dbl[])  [unwired: 3 in]
              "拟合参数" <- w306
              n135 = call "从动态数据转换2"("Dynamic Data Type"=w314) -> ("Array"=w277:dbl[])  [unwired: 3 in]
              n136 = Build Array(w273, w272, w282, w277, w306, w283) -> (w344:dbl[][])
              n137 = call-poly <vilib>:"Write Delimited Spreadsheet.vi"("file path (dialog if empty)"=w341, "format (%.3f)"="%.16f", "2D data"=w344, "append to file? (new file:F)"=TRUE ("append to file? (F)"), "transpose? (no:F)"=TRUE ("transpose? (F)")) -> ()  [unwired: 9 in, 2 out]
              n138 = Index Array(array=w306, index #1=0 ("索引"), index #2=1 ("索引")) -> (element #1=→"xc":dbl, element #2=w280:dbl)
              "w" <- w280
              n139 = Bundle("波长范围"=w285, "Filtered X"=w276) -> (w288:cluster{"波长范围 ":dbl[], "Filtered X":dbl[]})  [unwired: 1 in]
              n140 = Bundle(w289, "Array"=w277) -> (w287:cluster{dbl[], "Array":dbl[]})  [unwired: 1 in]
              n141 = Array Max & Min(array=w277) -> (max value=w274:dbl)  [unwired: 3 out]
              "拟合峰值" <- w274
              n142 = Array Max & Min(array=w276) -> (max value=w275:dbl)  [unwired: 3 out]
              "原始峰值" <- w275
              n143 = Build Array(w288, w287) -> (w286:cluster{"波长范围 ":dbl[], "Array":dbl[]}[])
              n144 = local write "best fit"(w286) -> ()
            }
            frame #7 {
              n145 = flat-sequence {
                tunnel: w369 -> [w378]
                tunnel: w368 -> [w377]
                tunnel: [w373] -> w367
                tunnel: [w372] -> w366
                frame #0 {
                  n146 = local read "channel输出口"() -> (w371:i32)
                  n147 = case shown="0, 默认" w371 {
                    tunnel: [1 0] -> w370
                    frame 0, Default {
                    }
                    frame 1 {
                    }
                  }
                  n148 = local write "Output 2"(TRUE ("布尔")) -> ()
                  n149 = Pick Line(multi-line string=":OUTP1 ON\n:OUTP2 ON" ("write buffer"), line index=w370) -> (output string=w374:string)  [unwired: 1 in]
                  n150 = VISA Write(VISA resource name=w378, write buffer=w374, error in (no error)=w377) -> (VISA resource name out=w373:refnum<visa-resource-name>, error out=w372:errorcluster)  [unwired: 1 out]
                }
              }
            }
            frame #8 {
              w381 = " \u0001\u0000¡"  # Channel
              n151 = Concatenate Strings(w381, "\r") -> (w387:string)
              n152 = VISA Write(VISA resource name=w383, write buffer=w387, error in (no error)=w386) -> (VISA resource name out=w385:refnum<visa-resource-name>, error out=w384:errorcluster)  [unwired: 1 out]
              n153 = local write "照明光"(TRUE ("照明光")) -> ()
            }
            frame #9 {
              n154 = Wait (ms)(milliseconds to wait=1200) -> ()  [unwired: 1 out]
            }
            frame #10 {
              n155 = Greater Or Equal?(x=w392, y=1) -> (x >= y?=w393:bool)
              n156 = case shown="真" w393 {
                tunnel: w395 -> [_ w401]
                tunnel: w394 -> [_ w402]
                tunnel: w390 -> [w396 w403]
                frame False {
                  n157 = local write "w0"(w396) -> ()
                }
                frame True {
                  n158 = local read "Δw1>C"() -> (w400:bool)
                  n159 = case shown="假" w400 {
                    tunnel: w403 -> [w422 w442]
                    tunnel: w402 -> [w412 _]
                    tunnel: w401 -> [w413 _]
                    frame False {
                      # "判断Δw突变位置并记录当前θ值"
                      # "根据θ变化速度改变开光时间"
                      n160 = local read "w0"() -> (w420:dbl)
                      n161 = Subtract(x=w413, y=w412) -> (x-y=w415:dbl)
                      n162 = local read "开光时间/ms"() -> (w418:u32)
                      n163 = Subtract(x=w420, y=w422) -> (x-y=w425:dbl)
                      n164 = Absolute Value(x=w415) -> (abs(x)=w417:dbl)
                      n165 = Absolute Value(x=w425) -> (abs(x)=w423:dbl)
                      n166 = Greater Or Equal?(x=w417, y=4.0) -> (x >= y?=w416:bool)
                      n167 = Greater Or Equal?(x=w423, y="C=w-w0") -> (x >= y?=w421:bool)
                      n168 = case shown="真" w421 {
                        tunnel: w412 -> [_ w440]
                        frame False {
                          w438 = FALSE ("Δw1>C")
                          n169 = local write "Δw1>C"(w438) -> ()
                          n170 = local write "Δw2>C"(w438) -> ()
                        }
                        frame True {
                          "θi" <- w440
                          "Δw1>C" <- TRUE ("布尔")
                        }
                      }
                      n171 = case shown="假" w416 {
                        tunnel: w417 -> [w430 _]
                        tunnel: w418 -> [w427 w437]
                        tunnel: [w426 w435] -> w419
                        frame False {
                          n172 = Less Or Equal?(x=w430, y=1.0) -> (x <= y?=w428:bool)
                          n173 = case shown="真" w428 {
                            tunnel: w427 -> [w431 w434]
                            tunnel: [w431 w433] -> w426
                            frame False {
                            }
                            frame True {
                              n174 = Multiply(x=w434, y="角度倍乘系数") -> (x*y=w433:dbl)
                            }
                          }
                        }
                        frame True {
                          n175 = Divide(x=w437, y=1.6) -> (x/y=w435:dbl)
                        }
                      }
                      n176 = local write "开光时间/ms"(w419) -> ()
                    }
                    frame True {
                      # "再次判断Δw，排除坏点影响"
                      n177 = local read "Δw2>C"() -> (w441:bool)
                      n178 = case shown="假" w441 {
                        tunnel: w442 -> [w447 _]
                        frame False {
                          n179 = local read "C=w-w0"() -> (w444:dbl)
                          n180 = local read "w0"() -> (w448:dbl)
                          n181 = Subtract(x=w448, y=w447) -> (x-y=w450:dbl)
                          n182 = Absolute Value(x=w450) -> (abs(x)=w449:dbl)
                          n183 = Add(x=w444, y=0.5) -> (x+y=w443:dbl)
                          n184 = Greater Or Equal?(x=w449, y=w443) -> (x >= y?=w446:bool)
                          n185 = case shown="真" w446 {
                            frame False {
                              n186 = local write "θi"(0.0 ("θi")) -> ()
                              n187 = local write "Δw1>C"(FALSE ("Δw1>C")) -> ()
                            }
                            frame True {
                              "Δw2>C" <- TRUE
                            }
                          }
                        }
                        frame True {
                        }
                      }
                    }
                  }
                  n188 = local read "Δw1>C"() -> (w398:bool)
                  n189 = local read "Δw2>C"() -> (w399:bool)
                  n190 = And(x=w398, y=w399) -> (x .and. y?=w397:bool)
                  n191 = case shown="真" w397 {
                    tunnel: w401 -> [_ w404]
                    frame False {
                    }
                    frame True {
                      # "4°后重置指示灯状态"
                      n192 = local read "θi"() -> (w408:dbl)
                      n193 = Subtract(x=w404, y=w408) -> (x-y=w409:dbl)
                      n194 = Absolute Value(x=w409) -> (abs(x)=w407:dbl)
                      n195 = Greater?(x=w407, y=4.0) -> (0:w405:bool)
                      n196 = case shown="真" w405 {
                        frame False {
                        }
                        frame True {
                          w410 = FALSE ("Δw1>C")
                          n197 = local write "Δw1>C"(w410) -> ()
                          n198 = local write "Δw2>C"(w410) -> ()
                          n199 = local write "θi"(0.0 ("θ")) -> ()
                        }
                      }
                    }
                  }
                }
              }
            }
            frame #11 {
              n200 = local write "正在测量"(FALSE) -> ()
            }
          }
          n201 = Build Array(w143, w142, w141, w140, w136) -> (w134:dbl[])
          n202 = local read "结果展示"() -> (w133:dbl[][])
          n203 = Insert Into Array(array=w133, new element=w134) -> (→"结果展示":dbl[][])  [unwired: 2 in]
        }
        n204 = Path To String(path=w97) -> (string=w106:string)
        n205 = Concatenate Strings(w106, "循环汇总" ("字符串"), ".xls" ("字符串")) -> (w105:string)
        n206 = VISA Close(VISA resource name=w121, error in (no error)=w120) -> (error out=→"output control error":errorcluster)
        n207 = VISA Close(VISA resource name=w124, error in (no error)=w123) -> (error out=→"照明光error out":errorcluster)
        n208 = String To Path(string=w105) -> (path=w104:path)
        n209 = call-poly <vilib>:"Write Delimited Spreadsheet.vi"("file path (dialog if empty)"=w104, "format (%.3f)"="%.16f", "2D data"=w100, "append to file? (new file:F)"=TRUE ("append to file? (F)"), "transpose? (no:F)"=FALSE ("transpose? (F)")) -> ()  [unwired: 9 in, 2 out]
        n210 = local write "结果展示"(dbl[][] [] ("结果展示")) -> ()
      }
    }
    n211 = event shown="[0] 超时" {
      selector: _ -> [_ _]
      dyn-events: _ -> [_ _]
      timeout: u32 0 ("Time") -> [_ _]
      tunnel: "低电平持续输出" -> [_ w484]
      event Timeout {
        n212 = event-data() -> ()  [unwired: 1 in, 2 out]
      }
      event "低电平持续输出": Value Change {
        w488 = " :SOUR1\n :SOUR2"  # Channel
        n213 = event-data() -> ()  [unwired: 1 in, 6 out]
        n214 = local read "channel输出口"() -> (w489:i32)
        n215 = Pick Line(multi-line string=w488, line index=w489) -> (output string=w487:string)  [unwired: 1 in]
        n216 = local read "VISA 信号发生器"() -> (w492:refnum<visa-resource-name>)
        n217 = VISA Open(VISA resource name=w492) -> (VISA resource name=w491:refnum<visa-resource-name>, error out=w490:errorcluster)  [unwired: 4 in]
        n218 = stacked-sequence {
          seq-local: [w498 _ _ _ _ _ _ _ _ _ _ _ _] -> [_ _ w513 _ _ _ _ _ _ _ _ _ _]
          seq-local: [w497 _ _ _ _ _ _ _ _ _ _ _ _] -> [_ _ w512 _ _ _ _ _ _ _ _ _ _]
          seq-local: [_ _ w511 _ _ _ _ _ _ _ _ _ _] -> [_ _ _ _ w516 _ _ _ _ _ _ _ _]
          seq-local: [_ _ w510 _ _ _ _ _ _ _ _ _ _] -> [_ _ _ _ w517 _ _ _ _ _ _ _ _]
          seq-local: [_ _ _ _ w525 _ _ _ _ _ _ _ _] -> [_ _ _ _ _ _ w536 _ _ _ _ _ _]
          seq-local: [_ _ _ _ w524 _ _ _ _ _ _ _ _] -> [_ _ _ _ _ _ w535 _ _ _ _ _ _]
          seq-local: [_ _ _ _ _ _ w529 _ _ _ _ _ _] -> [_ _ _ _ _ _ _ _ w539 _ _ _ _]
          seq-local: [_ _ _ _ _ _ w528 _ _ _ _ _ _] -> [_ _ _ _ _ _ _ _ w538 _ _ _ _]
          seq-local: [_ _ _ _ _ _ _ _ w542 _ _ _ _] -> [_ _ _ _ _ _ _ _ _ _ w553 _ _]
          seq-local: [_ _ _ _ _ _ _ _ w541 _ _ _ _] -> [_ _ _ _ _ _ _ _ _ _ w552 _ _]
          seq-local: [_ _ _ _ _ _ _ _ _ _ w550 _ _] -> [_ _ _ _ _ _ _ _ _ _ _ _ w567]
          seq-local: [_ _ _ _ _ _ _ _ _ _ w549 _ _] -> [_ _ _ _ _ _ _ _ _ _ _ _ w566]
          tunnel: w491 -> [w503 _ _ _ _ _ _ _ _ _ _ _ _]
          tunnel: w490 -> [w496 _ _ _ _ _ _ _ _ _ _ _ _]
          tunnel: w487 -> [w495 _ w509 _ w522 _ w533 _ w543 _ w556 _ _]
          tunnel: [_ _ _ _ _ _ _ _ _ _ _ _ w565] -> w486
          tunnel: [_ _ _ _ _ _ _ _ _ _ _ _ w563] -> w485
          tunnel: w484 -> [_ _ _ _ _ _ _ _ _ _ _ _ w564]
          frame #0 {
            w500 = " PULSe"  # Function Command
            n219 = local read "输出信号波形"() -> (w494:u16)
            n220 = Concatenate Strings(w495, ":FUNC" ("string (\"\")")) -> (w501:string)
            n221 = Pick Line(string ("")=w501, multi-line string=w500, line index=w494) -> (output string=w499:string)
            n222 = VISA Write(VISA resource name=w503, write buffer=w499, error in (no error)=w496) -> (VISA resource name out=w498:refnum<visa-resource-name>, error out=w497:errorcluster)  [unwired: 1 out]
          }
          frame #1 {
            n223 = Wait (ms)(milliseconds to wait=u32 150) -> ()  [unwired: 1 out]
          }
          frame #2 {
            n224 = Number To Fractional String(use system decimal point (T)=TRUE ("使用系统小数点(T)"), number=1.0 ("数字")) -> (F-format string=w507:string)  [unwired: 2 in]
            n225 = Concatenate Strings ("连接字符串")(w509, ":VOLTage：HIGH ", w507) -> (w506:string)
            n226 = VISA Write(VISA resource name=w513, write buffer=w506, error in (no error)=w512) -> (VISA resource name out=w511:refnum<visa-resource-name>, error out=w510:errorcluster)  [unwired: 1 out]
          }
          frame #3 {
            n227 = Wait (ms)(milliseconds to wait=u32 150) -> ()  [unwired: 1 out]
          }
          frame #4 {
            # "1 电压偏置"
            n228 = Number To Fractional String(use system decimal point (T)=TRUE ("使用系统小数点(T)"), number=0.0 ("数字")) -> (F-format string=w520:string)  [unwired: 2 in]
            n229 = Concatenate Strings(w522, ":VOLTage:LOW ", w520) -> (w521:string)
            n230 = VISA Write(VISA resource name=w516, write buffer=w521, error in (no error)=w517) -> (VISA resource name out=w525:refnum<visa-resource-name>, error out=w524:errorcluster)  [unwired: 1 out]
          }
          frame #5 {
            n231 = Wait (ms)(milliseconds to wait=u32 150) -> ()  [unwired: 1 out]
          }
          frame #6 {
            n232 = local read "channel输出口"() -> (w531:i32)
            n233 = Pick Line(multi-line string=":OUTP1:IMPedance \n:OUTP2:IMPedance " ("write buffer"), line index=w531) -> (output string=w530:string)  [unwired: 1 in]
            n234 = Concatenate Strings ("连接字符串")(w533, w530, "INFINITY") -> (w534:string)
            n235 = VISA Write(VISA resource name=w536, write buffer=w534, error in (no error)=w535) -> (VISA resource name out=w529:refnum<visa-resource-name>, error out=w528:errorcluster)  [unwired: 1 out]
          }
          frame #7 {
            n236 = Wait (ms)(milliseconds to wait=u32 150) -> ()  [unwired: 1 out]
          }
          frame #8 {
            n237 = Number To Fractional String(use system decimal point (T)=TRUE ("使用系统小数点(T)"), number=0.0 ("数字")) -> (F-format string=w546:string)  [unwired: 2 in]
            n238 = Concatenate Strings(w543, ":PULSe:DELay ", w546) -> (w544:string)
            n239 = VISA Write(VISA resource name=w539, write buffer=w544, error in (no error)=w538) -> (VISA resource name out=w542:refnum<visa-resource-name>, error out=w541:errorcluster)  [unwired: 1 out]
          }
          frame #9 {
            n240 = Wait (ms)(milliseconds to wait=u32 150) -> ()  [unwired: 1 out]
          }
          frame #10 {
            w557 = ":LEADing\n:TRAiling "  # Channel
            w561 = ":PULSe:TRANsition"  # VOLTage:Offset
            n241 = local read "上升下降沿"() -> (w558:i32)
            n242 = Pick Line(multi-line string=w557, line index=w558) -> (output string=w554:string)  [unwired: 1 in]
            n243 = Number To Fractional String(use system decimal point (T)=TRUE ("使用系统小数点(T)"), number=0.0 ("数字")) -> (F-format string=w555:string)  [unwired: 2 in]
            n244 = Concatenate Strings(w556, w561, w554, w555) -> (w559:string)
            n245 = VISA Write(VISA resource name=w553, write buffer=w559, error in (no error)=w552) -> (VISA resource name out=w550:refnum<visa-resource-name>, error out=w549:errorcluster)  [unwired: 1 out]
          }
          frame #11 {
            n246 = Wait (ms)(milliseconds to wait=u32 150) -> ()  [unwired: 1 out]
          }
          frame #12 {
            n247 = case shown="假" w564 {
              tunnel: w567 -> [w575 w576]
              tunnel: [w574 w583] -> w563
              tunnel: w566 -> [w573 w581]
              tunnel: [w572 w582] -> w565
              frame True {
                n248 = local write "Output"(TRUE ("布尔")) -> ()
                n249 = local read "channel输出口"() -> (w569:i32)
                n250 = Pick Line(multi-line string=":OUTP1 ON\n:OUTP2 ON" ("write buffer"), line index=w569) -> (output string=w568:string)  [unwired: 1 in]
                n251 = VISA Write(VISA resource name=w575, write buffer=w568, error in (no error)=w573) -> (VISA resource name out=w572:refnum<visa-resource-name>, error out=w574:errorcluster)  [unwired: 1 out]
              }
              frame False {
                n252 = local read "channel输出口"() -> (w578:i32)
                n253 = Pick Line(multi-line string=":OUTP1 OFF\n:OUTP2 OFF" ("write buffer"), line index=w578) -> (output string=w577:string)  [unwired: 1 in]
                n254 = VISA Write(VISA resource name=w576, write buffer=w577, error in (no error)=w581) -> (VISA resource name out=w582:refnum<visa-resource-name>, error out=w583:errorcluster)  [unwired: 1 out]
                n255 = local write "Output"(FALSE ("布尔")) -> ()
              }
            }
          }
        }
        n256 = VISA Close(VISA resource name=w486, error in (no error)=w485) -> (error out=→"output control error  4":errorcluster)
      }
    }
    n257 = event shown="[0] 超时" {
      selector: _ -> [_ _]
      dyn-events: _ -> [_ _]
      timeout: u32 0 ("Time") -> [_ _]
      tunnel: "Enable" -> [_ w459]
      event Timeout {
        n258 = event-data() -> ()  [unwired: 1 in, 2 out]
      }
      event "Enable": Value Change {
        n259 = event-data() -> ()  [unwired: 1 in, 6 out]
        n260 = local read "VISA 信号发生器"() -> (w455:refnum<visa-resource-name>)
        n261 = VISA Open(VISA resource name=w455) -> (VISA resource name=w458:refnum<visa-resource-name>, error out=w461:errorcluster)  [unwired: 4 in]
        n262 = stacked-sequence {
          tunnel: w459 -> [w466 _]
          tunnel: w461 -> [w465 _]
          tunnel: w458 -> [w464 _]
          tunnel: [w463 _] -> w457
          tunnel: [w462 _] -> w456
          frame #0 {
            n263 = case shown="真" w466 {
              tunnel: w464 -> [w474 w482]
              tunnel: [w473 w481] -> w462
              tunnel: w465 -> [w472 w479]
              tunnel: [w471 w480] -> w463
              frame True {
                n264 = local write "Output"(TRUE ("布尔")) -> ()
                n265 = local read "channel输出口"() -> (w468:i32)
                n266 = Pick Line(multi-line string=":OUTP1 ON\n:OUTP2 ON" ("write buffer"), line index=w468) -> (output string=w467:string)  [unwired: 1 in]
                n267 = VISA Write(VISA resource name=w474, write buffer=w467, error in (no error)=w472) -> (VISA resource name out=w471:refnum<visa-resource-name>, error out=w473:errorcluster)  [unwired: 1 out]
              }
              frame False {
                n268 = local read "channel输出口"() -> (w476:i32)
                n269 = Pick Line(multi-line string=":OUTP1 OFF\n:OUTP2 OFF" ("write buffer"), line index=w476) -> (output string=w475:string)  [unwired: 1 in]
                n270 = VISA Write(VISA resource name=w482, write buffer=w475, error in (no error)=w479) -> (VISA resource name out=w480:refnum<visa-resource-name>, error out=w481:errorcluster)  [unwired: 1 out]
                n271 = local write "Output"(FALSE ("布尔")) -> ()
              }
            }
          }
          frame #1 {
            n272 = Wait (ms)(milliseconds to wait=u32 150) -> ()  [unwired: 1 out]
          }
        }
        n273 = VISA Close(VISA resource name=w457, error in (no error)=w456) -> (error out=→"output control error  5":errorcluster)
      }
    }
    n274 = event shown="[0] 超时" {
      selector: _ -> [_ _]
      dyn-events: _ -> [_ _]
      timeout: u32 0 ("Time") -> [_ _]
      tunnel: "Enable 2" -> [_ w27]
      event Timeout {
        n275 = event-data() -> ()  [unwired: 1 in, 2 out]
      }
      event "Enable 2": Value Change {
        n276 = event-data() -> ()  [unwired: 1 in, 6 out]
        n277 = Not(x=w27) -> (.not. x?=w26:bool)
        n278 = local read "VISA 信号发生器"() -> (w28:refnum<visa-resource-name>)
        n279 = VISA Open(VISA resource name=w28) -> (VISA resource name=w31:refnum<visa-resource-name>, error out=w32:errorcluster)  [unwired: 4 in]
        n280 = stacked-sequence {
          tunnel: w26 -> [w37 _]
          tunnel: w32 -> [w36 _]
          tunnel: w31 -> [w35 _]
          tunnel: [w34 _] -> w30
          tunnel: [w33 _] -> w29
          frame #0 {
            n281 = case shown="真" w37 {
              tunnel: w35 -> [w46 w57]
              tunnel: [w45 w56] -> w33
              tunnel: w36 -> [w44 w54]
              tunnel: [w43 w55] -> w34
              frame True {
                n282 = local read "channel输出口"() -> (w39:i32)
                n283 = local write "Output 2"(FALSE ("布尔")) -> ()
                n284 = case shown="1" w39 {
                  tunnel: [1 0] -> w38
                  frame 0, Default {
                  }
                  frame 1 {
                  }
                }
                n285 = Pick Line(multi-line string=":OUTP1 ON\n:OUTP2 ON" ("write buffer"), line index=w38) -> (output string=w40:string)  [unwired: 1 in]
                n286 = VISA Write(VISA resource name=w46, write buffer=w40, error in (no error)=w44) -> (VISA resource name out=w43:refnum<visa-resource-name>, error out=w45:errorcluster)  [unwired: 1 out]
              }
              frame False {
                n287 = local read "channel输出口"() -> (w50:i32)
                n288 = case shown="1" w50 {
                  tunnel: [1 0] -> w49
                  frame 0, Default {
                  }
                  frame 1 {
                  }
                }
                n289 = Pick Line(multi-line string=":OUTP1 OFF\n:OUTP2 OFF" ("write buffer"), line index=w49) -> (output string=w51:string)  [unwired: 1 in]
                n290 = VISA Write(VISA resource name=w57, write buffer=w51, error in (no error)=w54) -> (VISA resource name out=w55:refnum<visa-resource-name>, error out=w56:errorcluster)  [unwired: 1 out]
                n291 = local write "Output 2"(TRUE ("布尔")) -> ()
              }
            }
          }
          frame #1 {
            n292 = Wait (ms)(milliseconds to wait=u32 150) -> ()  [unwired: 1 out]
          }
        }
        n293 = VISA Close(VISA resource name=w30, error in (no error)=w29) -> ()  [unwired: 1 out]
      }
    }
    n294 = case shown="假" "设置参数" {
      frame False {
      }
      frame True {
        w590 = " :SOUR1\n :SOUR2"  # Channel
        n295 = local read "VISA 信号发生器"() -> (w592:refnum<visa-resource-name>)
        n296 = local read "channel输出口"() -> (w591:i32)
        n297 = case shown="1" w591 {
          tunnel: [1 0] -> w584
          frame 0, Default {
          }
          frame 1 {
          }
        }
        n298 = VISA Open(VISA resource name=w592) -> (VISA resource name=w595:refnum<visa-resource-name>, error out=w596:errorcluster)  [unwired: 4 in]
        n299 = Pick Line(multi-line string=w590, line index=w584) -> (output string=w585:string)  [unwired: 1 in]
        n300 = Pick Line(multi-line string=w590, line index=w591) -> (output string=w593:string)  [unwired: 1 in]
        n301 = stacked-sequence {
          seq-local: [w692 _ _ _ _ _ _ _ _ _ _ _ _ _ _] -> [_ _ w707 _ _ _ _ _ _ _ _ _ _ _ _]
          seq-local: [w691 _ _ _ _ _ _ _ _ _ _ _ _ _ _] -> [_ _ w706 _ _ _ _ _ _ _ w745 _ _ _ _]
          seq-local: [_ _ w705 _ _ _ _ _ _ _ _ _ _ _ _] -> [_ _ _ _ w716 _ _ _ _ _ _ _ _ _ _]
          seq-local: [_ _ w704 _ _ _ _ _ _ _ _ _ _ _ _] -> [_ _ _ _ w715 _ _ _ _ _ _ _ _ _ _]
          seq-local: [_ _ _ _ w714 _ _ _ _ _ _ _ _ _ _] -> [_ _ _ _ _ _ w722 _ _ _ _ _ _ _ _]
          seq-local: [_ _ _ _ w711 _ _ _ _ _ _ _ _ _ _] -> [_ _ _ _ _ _ w721 _ _ _ _ _ _ _ _]
          seq-local: [_ _ _ _ _ _ w729 _ _ _ _ _ _ _ _] -> [_ _ _ _ _ _ _ _ w740 _ _ _ _ _ _]
          seq-local: [_ _ _ _ _ _ w728 _ _ _ _ _ _ _ _] -> [_ _ _ _ _ _ _ _ w739 _ _ _ _ _ _]
          seq-local: [_ _ _ _ _ _ _ _ w733 _ _ _ _ _ _] -> [_ _ _ _ _ _ _ _ _ _ w746 _ _ _ _]
          seq-local: [_ _ _ _ _ _ _ _ w732 _ _ _ _ _ _] -> [_ _ _ _ _ _ _ _ _ _ _ _ _ _ _]
          seq-local: [_ _ _ _ _ _ _ _ _ _ w742 _ _ _ _] -> [_ _ _ _ _ _ _ _ _ _ _ _ w756 _ _]
          seq-local: [_ _ _ _ _ _ _ _ _ _ w743 _ _ _ _] -> [_ _ _ _ _ _ _ _ _ _ _ _ w755 _ _]
          seq-local: [_ _ _ _ _ _ _ _ _ _ _ _ w754 _ _] -> [_ _ _ _ _ _ _ _ _ _ _ _ _ _ w767]
          seq-local: [_ _ _ _ _ _ _ _ _ _ _ _ w753 _ _] -> [_ _ _ _ _ _ _ _ _ _ _ _ _ _ w766]
          tunnel: w595 -> [w697 _ _ _ _ _ _ _ _ _ _ _ _ _ _]
          tunnel: w596 -> [w690 _ _ _ _ _ _ _ _ _ _ _ _ _ _]
          tunnel: w593 -> [w689 _ w703 _ w710 _ w726 _ w737 _ w747 _ w757 _ w770]
          tunnel: [_ _ _ _ _ _ _ _ _ _ _ _ _ _ w765] -> w589
          tunnel: [_ _ _ _ _ _ _ _ _ _ _ _ _ _ w764] -> w588
          frame #0 {
            w694 = " PULSe"  # Function Command
            n302 = local read "输出信号波形"() -> (w688:u16)
            n303 = Concatenate Strings(w689, ":FUNC" ("string (\"\")")) -> (w695:string)
            n304 = Pick Line(string ("")=w695, multi-line string=w694, line index=w688) -> (output string=w693:string)
            n305 = VISA Write(VISA resource name=w697, write buffer=w693, error in (no error)=w690) -> (VISA resource name out=w692:refnum<visa-resource-name>, error out=w691:errorcluster)  [unwired: 1 out]
          }
          frame #1 {
            n306 = Wait (ms)(milliseconds to wait=u32 150) -> ()  [unwired: 1 out]
          }
          frame #2 {
            n307 = Number To Fractional String(use system decimal point (T)=TRUE ("使用系统小数点(T)"), number="低电平/V") -> (F-format string=w701:string)  [unwired: 2 in]
            n308 = Concatenate Strings ("连接字符串")(w703, ":VOLTage:LOW ", w701) -> (w700:string)
            n309 = VISA Write(VISA resource name=w707, write buffer=w700, error in (no error)=w706) -> (VISA resource name out=w705:refnum<visa-resource-name>, error out=w704:errorcluster)  [unwired: 1 out]
          }
          frame #3 {
            n310 = Wait (ms)(milliseconds to wait=u32 150) -> ()  [unwired: 1 out]
          }
          frame #4 {
            # "1 频率"
            n311 = Concatenate Strings(w710, ":FREQ ") -> (w717:string)
            n312 = Format Into String ("格式化写入字符串")(initial string=w717, "频率/Hz") -> (resulting string=w718:string)  [unwired: 2 in, 1 out]
            n313 = VISA Write(VISA resource name=w716, write buffer=w718, error in (no error)=w715) -> (VISA resource name out=w714:refnum<visa-resource-name>, error out=w711:errorcluster)  [unwired: 1 out]
          }
          frame #5 {
            n314 = Wait (ms)(milliseconds to wait=u32 150) -> ()  [unwired: 1 out]
          }
          frame #6 {
            n315 = Number To Fractional String(use system decimal point (T)=TRUE ("使用系统小数点(T)"), number="高电平/V") -> (F-format string=w723:string)  [unwired: 2 in]
            n316 = Concatenate Strings(w726, ":VOLTage:HIGH ", w723) -> (w725:string)
            n317 = VISA Write(VISA resource name=w722, write buffer=w725, error in (no error)=w721) -> (VISA resource name out=w729:refnum<visa-resource-name>, error out=w728:errorcluster)  [unwired: 1 out]
          }
          frame #7 {
            n318 = Wait (ms)(milliseconds to wait=u32 150) -> ()  [unwired: 1 out]
          }
          frame #8 {
            n319 = local read "channel输出口"() -> (w735:i32)
            n320 = Pick Line(multi-line string=":OUTP1:IMPedance \n:OUTP2:IMPedance " ("write buffer"), line index=w735) -> (output string=w734:string)  [unwired: 1 in]
            n321 = Concatenate Strings ("连接字符串")(w737, w734, "INFINITY") -> (w738:string)
            n322 = VISA Write(VISA resource name=w740, write buffer=w738, error in (no error)=w739) -> (VISA resource name out=w733:refnum<visa-resource-name>, error out=w732:errorcluster)  [unwired: 1 out]
          }
          frame #9 {
            n323 = Wait (ms)(milliseconds to wait=u32 150) -> ()  [unwired: 1 out]
          }
          frame #10 {
            n324 = Number To Fractional String(use system decimal point (T)=TRUE ("使用系统小数点(T)"), number="占空比/%") -> (F-format string=w749:string)  [unwired: 2 in]
            n325 = Concatenate Strings(w747, ":PULSe:DCYCle ", w749) -> (w744:string)
            n326 = VISA Write(VISA resource name=w746, write buffer=w744, error in (no error)=w745) -> (VISA resource name out=w742:refnum<visa-resource-name>, error out=w743:errorcluster)  [unwired: 1 out]
          }
          frame #11 {
            n327 = Wait (ms)(milliseconds to wait=u32 150) -> ()  [unwired: 1 out]
          }
          frame #12 {
            n328 = Number To Fractional String(use system decimal point (T)=TRUE ("使用系统小数点(T)"), number="延时/s") -> (F-format string=w760:string)  [unwired: 2 in]
            n329 = Concatenate Strings(w757, ":PULSe:DELay ", w760) -> (w758:string)
            n330 = VISA Write(VISA resource name=w756, write buffer=w758, error in (no error)=w755) -> (VISA resource name out=w754:refnum<visa-resource-name>, error out=w753:errorcluster)  [unwired: 1 out]
          }
          frame #13 {
            n331 = Wait (ms)(milliseconds to wait=u32 150) -> ()  [unwired: 1 out]
          }
          frame #14 {
            w771 = ":LEADing\n:TRAiling "  # Channel
            w776 = ":PULSe:TRANsition"  # VOLTage:Offset
            n332 = local read "上升下降沿"() -> (w772:i32)
            n333 = Pick Line(multi-line string=w771, line index=w772) -> (output string=w768:string)  [unwired: 1 in]
            n334 = Number To Fractional String(use system decimal point (T)=TRUE ("使用系统小数点(T)"), number="上升下降沿/s") -> (F-format string=w769:string)  [unwired: 2 in]
            n335 = Concatenate Strings(w770, w776, w768, w769) -> (w773:string)
            n336 = VISA Write(VISA resource name=w767, write buffer=w773, error in (no error)=w766) -> (VISA resource name out=w765:refnum<visa-resource-name>, error out=w764:errorcluster)  [unwired: 1 out]
          }
        }
        n337 = stacked-sequence {
          seq-local: [w603 _ _ _ _ _ _ _ _ _ _ _ _ _ _] -> [_ _ w618 _ _ _ _ _ _ _ _ _ _ _ _]
          seq-local: [w602 _ _ _ _ _ _ _ _ _ _ _ _ _ _] -> [_ _ w617 _ _ _ _ _ _ _ w656 _ _ _ _]
          seq-local: [_ _ w616 _ _ _ _ _ _ _ _ _ _ _ _] -> [_ _ _ _ w627 _ _ _ _ _ _ _ _ _ _]
          seq-local: [_ _ w615 _ _ _ _ _ _ _ _ _ _ _ _] -> [_ _ _ _ w626 _ _ _ _ _ _ _ _ _ _]
          seq-local: [_ _ _ _ w625 _ _ _ _ _ _ _ _ _ _] -> [_ _ _ _ _ _ w633 _ _ _ _ _ _ _ _]
          seq-local: [_ _ _ _ w622 _ _ _ _ _ _ _ _ _ _] -> [_ _ _ _ _ _ w632 _ _ _ _ _ _ _ _]
          seq-local: [_ _ _ _ _ _ w640 _ _ _ _ _ _ _ _] -> [_ _ _ _ _ _ _ _ w651 _ _ _ _ _ _]
          seq-local: [_ _ _ _ _ _ w639 _ _ _ _ _ _ _ _] -> [_ _ _ _ _ _ _ _ w650 _ _ _ _ _ _]
          seq-local: [_ _ _ _ _ _ _ _ w645 _ _ _ _ _ _] -> [_ _ _ _ _ _ _ _ _ _ w657 _ _ _ _]
          seq-local: [_ _ _ _ _ _ _ _ w644 _ _ _ _ _ _] -> [_ _ _ _ _ _ _ _ _ _ _ _ _ _ _]
          seq-local: [_ _ _ _ _ _ _ _ _ _ w653 _ _ _ _] -> [_ _ _ _ _ _ _ _ _ _ _ _ w667 _ _]
          seq-local: [_ _ _ _ _ _ _ _ _ _ w654 _ _ _ _] -> [_ _ _ _ _ _ _ _ _ _ _ _ w666 _ _]
          seq-local: [_ _ _ _ _ _ _ _ _ _ _ _ w665 _ _] -> [_ _ _ _ _ _ _ _ _ _ _ _ _ _ w680]
          seq-local: [_ _ _ _ _ _ _ _ _ _ _ _ w664 _ _] -> [_ _ _ _ _ _ _ _ _ _ _ _ _ _ w679]
          tunnel: w589 -> [w608 _ _ _ _ _ _ _ _ _ _ _ _ _ _]
          tunnel: w588 -> [w601 _ _ _ _ _ _ _ _ _ _ _ _ _ _]
          tunnel: w585 -> [w600 _ w614 _ w621 _ w637 _ w648 _ w658 _ w668 _ w675]
          tunnel: [_ _ _ _ _ _ _ _ _ _ _ _ _ _ w678] -> w587
          tunnel: [_ _ _ _ _ _ _ _ _ _ _ _ _ _ w677] -> w586
          tunnel: w584 -> [_ _ _ _ _ _ _ _ w642 _ _ _ _ _ _]
          frame #0 {
            w605 = " PULSe"  # Function Command
            n338 = Concatenate Strings(w600, ":FUNC" ("string (\"\")")) -> (w606:string)
            n339 = Pick Line(string ("")=w606, multi-line string=w605, line index="输出信号波形 2") -> (output string=w604:string)
            n340 = VISA Write(VISA resource name=w608, write buffer=w604, error in (no error)=w601) -> (VISA resource name out=w603:refnum<visa-resource-name>, error out=w602:errorcluster)  [unwired: 1 out]
          }
          frame #1 {
            n341 = Wait (ms)(milliseconds to wait=u32 150) -> ()  [unwired: 1 out]
          }
          frame #2 {
            n342 = Number To Fractional String(use system decimal point (T)=TRUE ("使用系统小数点(T)"), number="低电平/V 2") -> (F-format string=w612:string)  [unwired: 2 in]
            n343 = Concatenate Strings ("连接字符串")(w614, ":VOLTage:LOW ", w612) -> (w611:string)
            n344 = VISA Write(VISA resource name=w618, write buffer=w611, error in (no error)=w617) -> (VISA resource name out=w616:refnum<visa-resource-name>, error out=w615:errorcluster)  [unwired: 1 out]
          }
          frame #3 {
            n345 = Wait (ms)(milliseconds to wait=u32 150) -> ()  [unwired: 1 out]
          }
          frame #4 {
            # "1 频率"
            n346 = Concatenate Strings(w621, ":FREQ ") -> (w628:string)
            n347 = Format Into String ("格式化写入字符串")(initial string=w628, "频率/Hz 2") -> (resulting string=w629:string)  [unwired: 2 in, 1 out]
            n348 = VISA Write(VISA resource name=w627, write buffer=w629, error in (no error)=w626) -> (VISA resource name out=w625:refnum<visa-resource-name>, error out=w622:errorcluster)  [unwired: 1 out]
          }
          frame #5 {
            n349 = Wait (ms)(milliseconds to wait=u32 150) -> ()  [unwired: 1 out]
          }
          frame #6 {
            n350 = Number To Fractional String(use system decimal point (T)=TRUE ("使用系统小数点(T)"), number="高电平/V 2") -> (F-format string=w634:string)  [unwired: 2 in]
            n351 = Concatenate Strings(w637, ":VOLTage:HIGH ", w634) -> (w636:string)
            n352 = VISA Write(VISA resource name=w633, write buffer=w636, error in (no error)=w632) -> (VISA resource name out=w640:refnum<visa-resource-name>, error out=w639:errorcluster)  [unwired: 1 out]
          }
          frame #7 {
            n353 = Wait (ms)(milliseconds to wait=u32 150) -> ()  [unwired: 1 out]
          }
          frame #8 {
            n354 = Pick Line(multi-line string=":OUTP1:IMPedance \n:OUTP2:IMPedance " ("write buffer"), line index=w642) -> (output string=w646:string)  [unwired: 1 in]
            n355 = Concatenate Strings ("连接字符串")(w648, w646, "INFINITY") -> (w649:string)
            n356 = VISA Write(VISA resource name=w651, write buffer=w649, error in (no error)=w650) -> (VISA resource name out=w645:refnum<visa-resource-name>, error out=w644:errorcluster)  [unwired: 1 out]
          }
          frame #9 {
            n357 = Wait (ms)(milliseconds to wait=u32 150) -> ()  [unwired: 1 out]
          }
          frame #10 {
            n358 = Number To Fractional String(use system decimal point (T)=TRUE ("使用系统小数点(T)"), number="占空比/% 2") -> (F-format string=w660:string)  [unwired: 2 in]
            n359 = Concatenate Strings(w658, ":PULSe:DCYCle ", w660) -> (w655:string)
            n360 = VISA Write(VISA resource name=w657, write buffer=w655, error in (no error)=w656) -> (VISA resource name out=w653:refnum<visa-resource-name>, error out=w654:errorcluster)  [unwired: 1 out]
          }
          frame #11 {
            n361 = Wait (ms)(milliseconds to wait=u32 150) -> ()  [unwired: 1 out]
          }
          frame #12 {
            n362 = Number To Fractional String(use system decimal point (T)=TRUE ("使用系统小数点(T)"), number="延时/s 2") -> (F-format string=w671:string)  [unwired: 2 in]
            n363 = Concatenate Strings(w668, ":PULSe:DELay ", w671) -> (w669:string)
            n364 = VISA Write(VISA resource name=w667, write buffer=w669, error in (no error)=w666) -> (VISA resource name out=w665:refnum<visa-resource-name>, error out=w664:errorcluster)  [unwired: 1 out]
          }
          frame #13 {
            n365 = Wait (ms)(milliseconds to wait=u32 150) -> ()  [unwired: 1 out]
          }
          frame #14 {
            w683 = ":LEADing\n:TRAiling "  # Channel
            w687 = ":PULSe:TRANsition"  # VOLTage:Offset
            n366 = Pick Line(multi-line string=w683, line index="上升下降沿 2") -> (output string=w681:string)  [unwired: 1 in]
            n367 = Number To Fractional String(use system decimal point (T)=TRUE ("使用系统小数点(T)"), number="上升下降沿/s 2") -> (F-format string=w682:string)  [unwired: 2 in]
            n368 = Concatenate Strings(w675, w687, w681, w682) -> (w684:string)
            n369 = VISA Write(VISA resource name=w680, write buffer=w684, error in (no error)=w679) -> (VISA resource name out=w678:refnum<visa-resource-name>, error out=w677:errorcluster)  [unwired: 1 out]
          }
        }
        n370 = VISA Close(VISA resource name=w587, error in (no error)=w586) -> (error out=→"configure error out":errorcluster)
      }
    }
    n371 = event shown="[0] 超时" {
      selector: _ -> [_ _]
      dyn-events: _ -> [_ _]
      timeout: 0 -> [_ _]
      tunnel: "照明光" -> [_ w61]
      event Timeout {
        n372 = event-data() -> ()  [unwired: 1 in, 3 out]
      }
      event "照明光": Value Change {
        n373 = event-data() -> ()  [unwired: 1 in, 6 out]
        n374 = local read "stop bits (10: 1 bit)"() -> (w74:u16)
        n375 = local read "parity (0:none)"() -> (w73:enum16{"None", "Odd", "Even", "Mark", "Space"})
        n376 = local read "照明光VISA"() -> (w70:refnum<visa-resource-name>)
        n377 = local read "baud rate"() -> (w71:u32)
        n378 = local read "data bits (8)"() -> (w72:u16)
        n379 = call-poly "VISA Configure Serial Port"("VISA resource name"=w70, "baud rate (9600)"=w71, "data bits (8)"=w72, "parity (0:none)"=w73, "stop bits (10: 1 bit)"=w74) -> ("VISA resource name out"=w67:refnum<visa-resource-name>, "error out"=w66:errorcluster)  [unwired: 9 in]
        n380 = call <vilib>:"Simple Error Handler.vi"("error in (no error)"=w66) -> ()  [unwired: 4 in, 5 out]
        n381 = VISA Open(access mode=0, error in (no error)=w66, VISA resource name=w67) -> (VISA resource name=w69:refnum<visa-resource-name>, error out=w68:errorcluster)  [unwired: 2 in]
        n382 = stacked-sequence {
          tunnel: w69 -> [w79]
          tunnel: w68 -> [w78]
          tunnel: [w77] -> w64
          tunnel: [w76] -> w65
          tunnel: w61 -> [w75]
          frame #0 {
            n383 = case shown="假" w75 {
              tunnel: w79 -> [w85 w95]
              tunnel: [w83 w94] -> w77
              tunnel: w78 -> [w84 w93]
              tunnel: [w82 w92] -> w76
              frame False {
                n384 = Concatenate Strings(" \u0001\u0001¢", "\r") -> (w86:string)
                n385 = VISA Write(VISA resource name=w85, write buffer=w86, error in (no error)=w84) -> (VISA resource name out=w83:refnum<visa-resource-name>, error out=w82:errorcluster)  [unwired: 1 out]
                n386 = Wait (ms)(milliseconds to wait=50) -> ()  [unwired: 1 out]
              }
              frame True {
                w88 = " \u0001\u0000¡"  # Channel
                n387 = Wait (ms)(milliseconds to wait=50) -> ()  [unwired: 1 out]
                n388 = Concatenate Strings(w88, "\r") -> (w89:string)
                n389 = VISA Write(VISA resource name=w95, write buffer=w89, error in (no error)=w93) -> (VISA resource name out=w94:refnum<visa-resource-name>, error out=w92:errorcluster)  [unwired: 1 out]
              }
            }
          }
        }
        n390 = VISA Close(VISA resource name=w64, error in (no error)=w65) -> (error out=w63:errorcluster)
        n391 = call <vilib>:"Simple Error Handler.vi"("error in (no error)"=w63) -> ()  [unwired: 4 in, 5 out]
      }
    }
  }
  n392 = flat-sequence {
    frame #0 {
      "Backlight" <- i32[][] [] ("Backlight")
    }
    frame #1 {
      w778 = FALSE
      # "删除背景光控件\n初始值设定"
      n393 = local write "cut backlight"(w778) -> ()
      "backlight" <- w778
    }
  }
  n394 = stacked-sequence {
    seq-local: [_ _ _ w799 _ _ _ _] -> [_ _ _ _ w817 w837 w845 w1082]
    seq-local: [_ _ _ w798 _ _ _ _] -> [_ _ _ _ w818 w838 w844 w1083]
    frame #0 {
      # "initialize all variables"
      n395 = property on="initialize" class="Bool"("Désactivé"=u8 0) -> ()  [unwired: 2 in, 2 out]
      n396 = property on="Acquire" class="Bool"("Visible"=FALSE) -> ()  [unwired: 2 in, 2 out]
      n397 = property on="Setup" class="Bool (严格)"("Visible"=FALSE) -> ()  [unwired: 2 in, 2 out]
      n398 = local write "indicator"("" ("indicator")) -> ()
      n399 = local write "initialized ?"(FALSE ("initialized ?")) -> ()
      n400 = local write "Continuous"(FALSE ("Continuous")) -> ()
      n401 = local write "Close"(FALSE ("Close")) -> ()
      n402 = property on="Device Name" class="Ring (严格)"("Désactivé"=u8 0) -> ()  [unwired: 2 in, 2 out]
      n403 = property on="Continuous" class="Bool (严格)"("Visible"=FALSE) -> ()  [unwired: 2 in, 2 out]
      n404 = local write "Commande tab"(T1."Settings" ("Commande tab")) -> ()
    }
    frame #1 {
      # "Read Uniq ID"
      n405 = stacked-sequence {
        frame #0 {
          n406 = call "read detector uniq-id.vi"() -> ("nbr of components"=w791:i32, "UniqueID"=w790:string[], "Name"=w789:string[])  [unwired: 4 out]
          n407 = for {
            N: w791 -> [_]
            tunnel: w790 -> [w793]
            tunnel: w789 -> [w792]
            n408 = property on="Device Name" class="Ring (严格)"("Chaînes []"=w792) -> ()  [unwired: 2 in, 2 out]
            n409 = property on="Uniques ID" class="Ring (严格)"("Chaînes []"=w793) -> ()  [unwired: 2 in, 2 out]
          }
        }
      }
    }
    frame #2 {
      n410 = while {
        stop <- "initialize" stop-if-true
        n411 = local read "Device Name"() -> (w796:u16)
        n412 = local write "Uniques ID"(w796) -> ()
        n413 = local read "Close"() -> (w794:bool)
        n414 = Stop(stop? (T)=w794) -> ()
        n415 = Wait Until Next ms Multiple(millisecond multiple=u32 100 ("n millisecondes")) -> ()  [unwired: 1 out]
      }
    }
    frame #3 {
      n416 = stacked-sequence {
        tunnel: [_ w806 _ _] -> w799
        tunnel: [_ w805 _ _] -> w798
        frame #0 {
          n417 = local write "indicator"("Initializing ..." ("indicator")) -> ()
        }
        frame #1 {
          n418 = local read "Uniques ID"() -> (w803:u16)
          n419 = property on="Uniques ID" class="Ring (严格)"() -> ("Chaînes []"=w804:string[])  [unwired: 2 in, 2 out]
          n420 = Index Array(array=w804, index=w803) -> (element=w802:string)
          n421 = call "Initialize CCD.vi"("Unique id:"=w802) -> ("activeYPixels"=→"Y Pixels:":i32, "JYCCDLib.IJYCCDReqd"=w805:refnum<k7>, "activeXPixels"=→"X Pixels:":i32, "sortie d'erreur"=w806:errorcluster, "FirmwareVersion"=→"Firmware\nVersion":string)  [unwired: 3 out]
        }
        frame #2 {
          n422 = property on="initialize" class="Bool"("Désactivé"=u8 2) -> ()  [unwired: 2 in, 2 out]
          n423 = property on="Device Name" class="Ring (严格)"("Désactivé"=u8 2) -> ()  [unwired: 2 in, 2 out]
          n424 = local write "Continuous"(FALSE ("Continuous")) -> ()
          n425 = property on="Setup" class="Bool (严格)"("Visible"=TRUE) -> ()  [unwired: 2 in, 2 out]
        }
        frame #3 {
          n426 = local write "initialized ?"(TRUE ("initialized ?")) -> ()
          n427 = local write "indicator"("Initialized !" ("indicator")) -> ()
        }
      }
    }
    frame #4 {
      # "Actually not working"
      # "Read ADC and GAIN"
      n428 = case shown="假" "Constante de condition\n(Voir l'aide contextuelle)" {
        tunnel: w818 -> [_ w828]
        tunnel: w817 -> [_ w827]
        frame False {
        }
        frame True {
          # "Read Input supported trigger"
          n429 = call "Trigger - Get Supported Input.vi"("JYCCDLib.IJYCCDReqd"=w828, "Error Input"=w827) -> ("trigAddress"=w822:i32, "eventPtr"=w823:i32, "trigEventString"=w826:string, "trigSigType"=w825:i32, "trigSigTypeString"=w824:string)  [unwired: 4 out]
          n430 = local write "trigSigTypeString"(w824) -> ()
          n431 = local write "trigAddress"(w822) -> ()
          n432 = local write "Trigger Type :"(w823) -> ()
          n433 = local write "trigEventString"(w826) -> ()
          n434 = local write "Signal type :"(w825) -> ()
        }
      }
      n435 = call "Init ADC & Gain.vi"("JYCCDLib.IJYCCDReqd"=w818, "input error"=w817) -> ("ADC Number"=w816:i32[], "ADC description"=w821:string[], "Gain Number"=w819:i32[], "Gain description"=w820:string[])
      n436 = local write "Gain Number"(w819) -> ()
      n437 = local write "ADC Number"(w816) -> ()
      n438 = stacked-sequence {
        tunnel: w821 -> [w829 _]
        tunnel: w820 -> [_ w830]
        frame #0 {
          n439 = property on="ADC" class="Ring (严格)"("Chaînes []"=w829) -> ()  [unwired: 2 in, 2 out]
        }
        frame #1 {
          n440 = property on="GAIN" class="Ring (严格)"("Chaînes []"=w830) -> ()  [unwired: 2 in, 2 out]
        }
      }
    }
    frame #5 {
      # "IS multi Accumulation Supported ?"
      n441 = call "MultiAccu - Is Supported.vi"("Error In"=w837, "JYCCDLib.IJYCCDReqd"=w838) -> ("IsOperatingModeSupported"=w831:bool)  [unwired: 3 out]
      n442 = Select(t=0, s=w831, f=2) -> (s? t:f=w834:i32)
      n443 = Select(t=FALSE, s=w831, f=w831) -> (s? t:f=w833:bool)
      n444 = local write "Multi Accumulation mode:"(w833) -> ()
      n445 = property on="Multi Accumulation mode:" class="Bool (严格)"("Désactivé"=w834) -> ()  [unwired: 2 in, 2 out]
      n446 = property on="Multi Accumulation mode:" class="Bool (严格)"("Désactivé"=w834) -> ()  [unwired: 2 in, 2 out]
    }
    frame #6 {
      n447 = TCP Open Connection(address="地址", remote port or service name="端口") -> (connection ID=w841:refnum<k5>)  [unwired: 3 in, 1 out]
      n448 = while {
        tunnel: w844 -> [w870]
        tunnel: w845 -> [w869]
        tunnel: w841 -> [w852]
        shift-right: [w855] -> _
        shift-left: FALSE -> [w854]
        tunnel: [w846] -> w839
        stop <- "Close" stop-if-true
        n449 = local read "Continuous"() -> (w871:bool)
        n450 = Not(x=w854) -> (.not. x?=w856:bool)
        n451 = case shown="真" "Reformat" {
          frame False {
          }
          frame True {
            n452 = local read "Y Pixels:"() -> (w1057:i32)
            n453 = local read "X Pixels:"() -> (w1059:i32)
            n454 = call "Spectral Reformat CCD area.vi"("Y Pixels:"=w1057, "X Pixels:"=w1059, "numAreas"="Number of Areas :") -> ("areas :"=→"areas :":i32[][])  [unwired: 3 out]
          }
        }
        n455 = local read "Accumulations:"() -> (w866:u16)
        n456 = And(x="Setup", y=w856) -> (x .and. y?=w850:bool)
        n457 = case shown="真" w850 {
          tunnel: w852 -> [w876 w878]
          tunnel: [w876 w877] -> w851
          frame False {
          }
          frame True {
            n458 = TCP Write(connection ID=w878, data in="READY\\n") -> (connection ID out=w877:refnum<k5>)  [unwired: 2 in, 2 out]
          }
        }
        n459 = TCP Read(connection ID=w851, bytes to read="读取的字节", 9:"超时毫秒(25000)") -> (connection ID out=w858:refnum<k5>, data out=w862:string, error out=→"错误输出":errorcluster)  [unwired: 2 in]
        n460 = call <vilib>:"Trim Whitespace.vi"("string"=w862) -> ("trimmed string"=w863:string)  [unwired: 1 in]
        n461 = Equal?(x=w863, y="MEASURE") -> (x = y?=w849:bool)
        n462 = Or(x="Acquire", y=w849) -> (x .or. y?=w847:bool)
        n463 = Or(x=w847, y=w871) -> (x .or. y?=w868:bool)
        n464 = case shown="真" w868 {
          tunnel: w870 -> [_ w888]
          tunnel: w869 -> [_ w887]
          tunnel: "Enable InputTriggers :" -> [_ w886]
          tunnel: "Multi Accumulation mode:" -> [_ w885]
          tunnel: w866 -> [_ w884]
          tunnel: "MultiAcqShutterMode" -> [_ w883]
          tunnel: w858 -> [w880 w882]
          tunnel: [w880 w881] -> w846
          frame False {
          }
          frame True {
            n465 = stacked-sequence {
              seq-local: [_ _ w901 _ _] -> [_ _ _ w982 _]
              seq-local: [_ _ _ w948 _] -> [_ _ _ _ w1023]
              tunnel: w888 -> [_ w890 w905 w981 _]
              tunnel: w887 -> [_ w891 w904 w980 _]
              tunnel: w886 -> [_ w892 _ _ _]
              tunnel: w885 -> [_ _ w903 _ _]
              tunnel: w884 -> [_ _ w902 _ _]
              tunnel: w883 -> [_ _ w900 _ _]
              tunnel: w882 -> [_ _ _ w951 _]
              tunnel: [_ _ _ w940 _] -> w881
              frame #0 {
                n466 = local write "CCD Busy"(TRUE ("CCD Busy")) -> ()
              }
              frame #1 {
                n467 = case shown="假" w892 {
                  tunnel: w891 -> [w893 w899]
                  tunnel: w890 -> [w894 w898]
                  frame False {
                    n468 = call "Trigger - Disable.vi"("Error In"=w893, "JYCCDLib.IJYCCDReqd"=w894) -> ()  [unwired: 6 out]
                  }
                  frame True {
                    n469 = local read "Trigger Type :"() -> (w895:u16)
                    n470 = local read "Signal type :"() -> (w896:enum16{"TTL Rising Edge", "TTL Falling Edge"})
                    n471 = local read "trigAddress"() -> (w897:i32)
                    n472 = call "Trigger - Enable.vi"("Error In"=w899, "sigType"=w896, "event"=w895, "trigAddress"=w897, "JYCCDLib.IJYCCDReqd"=w898) -> ()  [unwired: 3 out]
                  }
                }
              }
              frame #2 {
                n473 = case shown="假" w903 {
                  selector: w903 -> [_ w934]
                  tunnel: w905 -> [w931 w937]
                  tunnel: w904 -> [w930 w936]
                  tunnel: w902 -> [_ w935]
                  tunnel: [u16 1 ("Accumulations:") w935] -> w901
                  tunnel: w900 -> [_ w933]
                  frame False {
                    n474 = call "MultiAccu - Disable.vi"("Error In"=w930, "JYCCDLib.IJYCCDReqd"=w931) -> ()  [unwired: 4 out]
                  }
                  frame True {
                    n475 = call "MultiAccu - Configure.vi"("JYCCDLib.IJYCCDReqd"=w937, "Cleans Before"="Number of Cleans", "Accumulations:"=w935, "MultiAcqHardwareMode"=w934, "MultiAcqShutterMode"=w933, "Error In"=w936) -> ()  [unwired: 1 in, 9 out]
                  }
                }
                n476 = flat-sequence {
                  frame #0 {
                    n477 = Current VI's Path() -> (path=w912:path)
                    n478 = Get Date/Time In Seconds() -> (seconds since 1Jan1904=w914:timestamp)
                    n479 = Strip Path(path=w912) -> (stripped path=w913:path)  [unwired: 1 out]
                    n480 = Path To String(path=w913) -> (string=w906:string)
                    n481 = Format Date/Time String(time format string (%c)="%m.%d" ("时间格式字符串(%c)"), seconds (now)=w914) -> (date/time string=w920:string)  [unwired: 1 in]
                    n482 = Concatenate Strings(w906, "\\Save\\" ("字符串"), w920) -> (w915:string)
                    n483 = String To Path(string=w915) -> (path=w916:path)
                    n484 = call <vilib>:"Check if File or Folder Exists.vi"("path"=w916) -> ("file or folder exists?"=w917:bool, "dup path"=w919:path)  [unwired: 8 in, 1 out]
                    n485 = case shown="真" w917 {
                      tunnel: [w927 w928] -> w918
                      tunnel: w919 -> [w926 w928]
                      tunnel: w920 -> [w925 _]
                      frame False {
                        n486 = Create Folder(prompt (Create Folder)=w925, path (use dialog)=w926) -> (created path=w927:path)  [unwired: 1 in, 2 out]
                      }
                      frame True {
                      }
                    }
                    n487 = Format Date/Time String(time format string (%c)="%y%m%d%H%M%S " ("时间格式字符串(%c)"), seconds (now)=w914) -> (date/time string=w923:string)  [unwired: 1 in]
                    n488 = Path To String(path=w918) -> (string=w921:string)
                    n489 = Concatenate Strings(w921, "\\" ("字符串")) -> (w922:string)
                    n490 = Concatenate Strings(w922, w923) -> (w911:string)
                    n491 = String To Path(string=w911) -> (path=→"最终存储路径 2":path)
                  }
                }
              }
              frame #3 {
                n492 = local read "cut backlight"() -> (w970:bool)
                n493 = local read "backlight"() -> (w969:bool)
                n494 = call "MultiAccu - Acquire spectral.vi"("error in"=w980, "Accumulations:"=w982, "ShutterOpen"="ShutterOpen", "JYCCDLib.IJYCCDReqd"=w981) -> ("Acq Time(ms)"=→"Acq Time(ms)":u32, "Array Out"=w979:i32[][][])  [unwired: 1 out]
                n495 = And(x=w970, y=w969) -> (x .and. y?=w971:bool)
                n496 = call "Array reset dimension.vi"("Area Number"="Area Number to Display", "Array In"=w979) -> ("Array Out"=w945:i32[][])
                n497 = case shown="假" w971 {
                  tunnel: [w1019 w1020] -> w972
                  tunnel: w945 -> [w1019 w1021]
                  frame False {
                  }
                  frame True {
                    n498 = local read "Backlight"() -> (w1022:i32[][])
                    n499 = Subtract(x=w1021, y=w1022) -> (x-y=w1020:i32[][])
                  }
                }
                n500 = local read "波长范围"() -> (w946:dbl[])
                n501 = local write "Data"(w945) -> ()
                n502 = Index Array(array=w972, index (row)=0 ("禁用的索引 (列)")) -> (element=w973:i32[])  [unwired: 1 in]
                n503 = Reverse 1D Array(array=w973) -> (reversed array=w938:i32[])
                n504 = Array To Spreadsheet String(delimiter (Tab)="分隔符(Tab)", array=w938, 3:"格式字符串") -> (spreadsheet string=w947:string)
                n505 = Concatenate Strings("DATA,", w947, "\\n") -> (w950:string)
                n506 = TCP Write(connection ID=w951, data in=w950) -> (connection ID out=w940:refnum<k5>)  [unwired: 2 in, 2 out]
                n507 = call "转换至动态数据2"("Array"=w946) -> ("Dynamic Data Type"=w975:dynamicdata)  [unwired: 3 in]
                n508 = call "转换至动态数据"("Array"=w938) -> ("Dynamic Data Type"=w976:dynamicdata)  [unwired: 3 in]
                n509 = call <vilib>:"Median Filter.vi"("left rank"=6, "X"=w938) -> ("Filtered X"=w963:dbl[])  [unwired: 8 in, 1 out]
                n510 = call "Build XY Graph2"("Y Input"=w976, "X Input"=w975) -> ("XY Graph"=w974:cluster{"Y":dbl[], "Y":dbl[]}[])  [unwired: 8 in, 1 out]
                n511 = Subtract(x="拟合终点", y="拟合起点") -> (x-y=w956:i32)
                n512 = local read "滤波阈值"() -> (w967:dbl)
                n513 = Array Subset(array=w946, index="拟合起点", length=w956) -> (w942:dbl[])
                n514 = local write "Spectrum"(w974) -> ()
                n515 = local read "拟合参数"() -> (w954:dbl[])
                n516 = In Range and Coerce(upper limit=w967, x=w963, lower limit=-100.0) -> (In Range?=w966:bool[])  [unwired: 1 out]
                n517 = Not(x=w966) -> (.not. x?=w960:bool[])
                n518 = local read "滤波阈值"() -> (w962:dbl)
                n519 = local write "范围内？"(w966) -> ()
                n520 = local read "X Pixels:"() -> (w964:i32)
                n521 = Or Array Elements(Boolean array=w960) -> (logical OR=w965:bool)
                n522 = case shown="假" w965 {
                  tunnel: w964 -> [_ w1006]
                  tunnel: w963 -> [w1002 w1005]
                  tunnel: [w1002 w1004] -> w944
                  tunnel: w962 -> [_ w1003]
                  frame False {
                  }
                  frame True {
                    n523 = for {
                      N: w1006 -> [_]
                      tunnel: w1005 -> [w1010] mode=indexing
                      tunnel: [w1009] -> w1004 mode=indexing
                      shift-right: [w1009] -> _
                      shift-left: _ -> [w1008]
                      tunnel: w1003 -> [w1007]
                      n524 = Greater?(x=w1010, y=w1007) -> (0:w1012:bool)
                      n525 = Less?(x=w1010, y=-100.0) -> (x < y?=w1013:bool)
                      n526 = Or(x=w1012, y=w1013) -> (x .or. y?=w1011:bool)
                      n527 = case shown="真" w1011 {
                        tunnel: w1010 -> [w1015 _]
                        tunnel: [w1015 w1017] -> w1009
                        tunnel: w1008 -> [_ w1018]
                        frame False {
                        }
                        frame True {
                          n528 = call <vilib>:"Median Filter PtByPt.vi"("rank"=5, "x"=w1018) -> ("Filtered x"=w1017:dbl)  [unwired: 2 in, 1 out]
                        }
                      }
                    }
                  }
                }
                n529 = Array Subset(array=w944, index="拟合起点", length=w956) -> (w943:dbl[])
                n530 = Bundle("波长范围"=w946, "Filtered X"=w944) -> (w955:cluster{"波长范围 ":dbl[], "Filtered X":dbl[]})  [unwired: 1 in]
                n531 = case shown="真" "是否拟合" {
                  tunnel: w943 -> [w985 w992]
                  tunnel: w942 -> [_ w987]
                  tunnel: [w985 w988] -> w939
                  tunnel: w955 -> [_ w990]
                  frame False {
                  }
                  frame True {
                    n532 = call "转换至动态数据7"("Array"=w992) -> ("Dynamic Data Type"=w997:dynamicdata)  [unwired: 3 in]
                    n533 = call "转换至动态数据8"("Array"=w987) -> ("Dynamic Data Type"=w998:dynamicdata)  [unwired: 3 in]
                    n534 = call "曲线拟合2"("Locations"=w998, "Signals"=w997) -> ("error out"=→"error out 2":errorcluster, "best fit"=w995:dynamicdata, "non-linear coefficients"=w996:dynamicdata)  [unwired: 5 in, 2 out]
                    n535 = call "从动态数据转换3"("Dynamic Data Type"=w996) -> ("Array"=w999:dbl[])  [unwired: 3 in]
                    n536 = call "从动态数据转换4"("Dynamic Data Type"=w995) -> ("Array"=w988:dbl[])  [unwired: 3 in]
                    n537 = local write "拟合参数"(w999) -> ()
                    n538 = Index Array(array=w999, index #1=0 ("索引"), index #2=1 ("索引")) -> (element #1=w1001:dbl, element #2=w1000:dbl)
                    n539 = local write "xc"(w1001) -> ()
                    n540 = Bundle(w987, "Array"=w988) -> (w991:cluster{dbl[], "Array":dbl[]})  [unwired: 1 in]
                    n541 = local write "w"(w1000) -> ()
                    n542 = Build Array(w990, w991) -> (→"best fit":cluster{"波长范围 ":dbl[], "Array":dbl[]}[])
                  }
                }
                n543 = Build Array(w942, w938, w939, w954) -> (w948:dbl[][])
              }
              frame #4 {
                n544 = case shown="真" "是否保存" {
                  tunnel: w1023 -> [_ w1028]
                  frame False {
                  }
                  frame True {
                    n545 = Get Date/Time In Seconds() -> (seconds since 1Jan1904=w1041:timestamp)
                    n546 = Get Date/Time String(date format (0)=enum16{"short", "long", "abbreviated"}."abbreviated" ("日期格式(0)"), seconds (now)=w1041, want seconds? (F)=TRUE ("需要秒？(F)")) -> (date string=w1039:string, time string=w1040:string)
                    n547 = Search and Replace String(replace all?=TRUE ("替换全部？(F)"), input string=w1040, search string=":" ("搜索字符串"), replace string="-" ("替换字符串(\"\")")) -> (result string=w1038:string)  [unwired: 4 in, 3 out]
                    n548 = local read "最终存储路径 2"() -> (w1042:path)
                    n549 = Path To String(path=w1042) -> (string=w1045:string)
                    n550 = Concatenate Strings(w1045, w1039, w1038, "光谱" ("字符串"), ".xls" ("字符串")) -> (w1044:string)
                    n551 = String To Path(string=w1044) -> (path=w1043:path)
                    n552 = call-poly <vilib>:"Write Delimited Spreadsheet.vi"("file path (dialog if empty)"=w1043, "format (%.3f)"="%.16f", "2D data"=w1028, "append to file? (new file:F)"=TRUE ("append to file? (F)"), "transpose? (no:F)"=TRUE ("transpose? (F)")) -> ()  [unwired: 9 in, 2 out]
                  }
                }
                n553 = case shown="假" "Save Backlight" {
                  frame False {
                  }
                  frame True {
                    w1046 = TRUE ("删除背景光")
                    n554 = local read "Data"() -> (w1048:i32[][])
                    n555 = local write "Backlight"(w1048) -> ()
                    n556 = local write "cut backlight"(w1046) -> ()
                    n557 = local write "backlight"(w1046) -> ()
                    n558 = local write "Save Backlight"(FALSE ("Save Backlight")) -> ()
                  }
                }
                n559 = local write "CCD Busy"(FALSE ("CCD Busy")) -> ()
              }
            }
          }
        }
        n560 = case shown="真" "Setup" {
          tunnel: w869 -> [_ w1064]
          tunnel: w870 -> [_ w1063]
          tunnel: [w1061 w1062] -> w855
          tunnel: w854 -> [w1061 _]
          frame False {
          }
          frame True {
            n561 = stacked-sequence {
              tunnel: w1064 -> [_ w1078 _]
              tunnel: w1063 -> [_ w1066 _]
              tunnel: [_ _ TRUE] -> w1062
              frame #0 {
                n562 = local write "indicator"("Setting up the detector" ("indicator")) -> ()
              }
              frame #1 {
                w1076 = 1 items=["JYMCD_ACQ_FORMAT_IMAGE", "JYMCD_ACQ_FORMAT_SCAN"] ("Acquisition type")
                n563 = local read "Gain Number"() -> (w1071:i32[])
                n564 = local read "GAIN"() -> (w1067:u16)
                n565 = local read "ADC Number"() -> (w1072:i32[])
                n566 = local read "ADC"() -> (w1068:u16)
                n567 = Index Array(array=w1071, index=w1067) -> (element=w1069:i32)
                n568 = Index Array(array=w1072, index=w1068) -> (element=w1070:i32)
                n569 = local read "Number of Areas :"() -> (w1074:u16)
                n570 = local read "areas :"() -> (w1075:i32[][])
                n571 = call "Setup CCD.vi"("numAreas"=w1074, "areas :"=w1075, "JYCCDLib.IJYCCDReqd"=w1066, "entrée d'erreur (pas d'erreur)"=w1078, "Acquisition type"=w1076, "Gain"=w1069, "Select ADC"=w1070, "Integration time(ms)"="Integration time (ms) :") -> ("DataSize"=→"DataSize":i32)  [unwired: 1 out]
                "JYCCDLib.IJYCCDReqd" <- w1066
              }
              frame #2 {
                w1080 = TRUE ("Visible")
                n572 = property on="Continuous" class="Bool (严格)"("Visible"=w1080) -> ()  [unwired: 2 in, 2 out]
                n573 = property on="Acquire" class="Bool"("Visible"=w1080) -> ()  [unwired: 2 in, 2 out]
                n574 = local write "indicator"("Ready !" ("indicator")) -> ()
              }
            }
          }
        }
        n575 = case shown="假" "Temperature" {
          tunnel: w870 -> [_ w1051]
          tunnel: w869 -> [_ w1050]
          frame False {
            n576 = property on="temp graph" class="WFChart (严格)"("Visible"=FALSE) -> ()  [unwired: 2 in, 2 out]
          }
          frame True {
            n577 = stacked-sequence {
              tunnel: w1051 -> [_ w1056]
              tunnel: w1050 -> [_ w1055]
              frame #0 {
                n578 = property on="temp graph" class="WFChart (严格)"("Visible"=TRUE) -> ()  [unwired: 2 in, 2 out]
              }
              frame #1 {
                w1054 = u16 0 items=["° Celsius", "Kelvin", "° Farenheit"] ("units")
                n579 = call "read temperature.vi"("entrée d'erreur (pas d'erreur)"=w1055, "units"=w1054, "JYCCDLib.IJYCCDReqd"=w1056) -> ("Current Temperature"=w1053:dbl)
                n580 = local write "temp graph"(w1053) -> ()
              }
            }
          }
        }
        n581 = Wait Until Next ms Multiple(millisecond multiple=u32 50 ("n millisecondes")) -> ()  [unwired: 1 out]
      }
      n582 = TCP Close Connection(connection ID=w839) -> ()  [unwired: 2 in, 2 out]
    }
    frame #7 {
      n583 = Close Reference(reference=w1083, error in (no error)=w1082) -> ()  [unwired: 1 out]
    }
  }
  n584 = stacked-sequence {
    seq-local: [_ _ w1093 _ _] -> [_ _ _ w1103 w1108]
    seq-local: [_ _ w1092 _ _] -> [_ _ _ w1102 _]
    seq-local: [_ _ _ w1101 _] -> [_ _ _ _ _]
    frame #0 {
      n585 = call "Get Monos From Config Browser.vi"() -> ("UniqueIDs"=w1088:string[], "Mono ID"=w1089:string[])  [unwired: 3 in, 1 out]
      n586 = Build Cluster Array(w1089, w1088) -> (w1086:cluster{"String":string, "String":string}[])
      n587 = property on="Mono ID" class="CmbBox"("Strings And Values []"=w1086) -> ()  [unwired: 2 in, 2 out]
      n588 = Index Array(array=w1086, index=0) -> (element=w1087:cluster{"String":string, "String":string})
      n589 = Unbundle(w1087) -> ("String"=w1084:string)  [unwired: 1 out]
      "Current UniqueID" <- w1084
      n590 = local write "Mono ID"(w1084) -> ()
    }
    frame #1 {
      n591 = while {
        stop <- "Connect" stop-if-true
        n592 = local read "Mono ID"() -> (w1090:string)
        n593 = local write "Current UniqueID"(w1090) -> ()
      }
    }
    frame #2 {
      n594 = local read "Mono ID"() -> (w1095:string)
      n595 = call "JYInitMono.vi"("Unique ID"=w1095, "Force Init"="Force\nInitialization") -> ("Refnum out"=w1093:refnum<k7>, "Initialized"=→"Initialized JY":bool, "error out"=w1092:errorcluster)  [unwired: 9 in, 2 out]
    }
    frame #3 {
      n596 = call "Show Current Grating.vi"("Refnum in"=w1103, "error in (no error)"=w1102) -> ("Gratings"=w1104:dbl[], "Grating Index"=w1098:i32, "Current Grating"=w1100:dbl, "Current Description"=w1097:string, "error out"=w1101:errorcluster)  [unwired: 5 in, 4 out]
      "Gratings" <- w1104
      n597 = local write "Current Grating"(w1100) -> ()
      n598 = local write "Current Description"(w1097) -> ()
      n599 = Number To Decimal String(number=w1104) -> (decimal integer string=w1106:string[])  [unwired: 1 in]
      n600 = Number To Decimal String(number=w1098) -> (decimal integer string=w1099:string)  [unwired: 1 in]
      n601 = property on="Target Grating" class="CmbBox"("Value"=w1099) -> ()  [unwired: 2 in, 2 out]
      n602 = Build Cluster Array(w1106, string[] ["1", "2", "3"]) -> (w1107:cluster{"Numeric":string, string}[])
      n603 = property on="Target Grating" class="CmbBox"("Strings And Values []"=w1107) -> ()  [unwired: 2 in, 2 out]
    }
    frame #4 {
      n604 = while {
        tunnel: w1108 -> [w1110]
        stop <- w1109 stop-if-true
        n605 = stacked-sequence {
          seq-local: [w1114 _ _ _ _] -> [_ w1121 w1132 _ w1140]
          seq-local: [w1113 _ _ _ _] -> [_ w1120 w1131 _ _]
          seq-local: [_ w1119 _ _ _] -> [_ _ _ _ _]
          seq-local: [_ w1118 _ _ _] -> [_ _ _ _ _]
          seq-local: [_ _ w1124 _ _] -> [_ _ _ _ _]
          seq-local: [_ _ w1123 _ _] -> [_ _ _ w1134 _]
          tunnel: w1110 -> [w1112 _ _ w1135 _]
          frame #0 {
            n606 = call "Show Current Grating.vi"("Refnum in"=w1112) -> ("Grating Index"=→"Grating Index":i32, "Current Grating"=→"Current Grating":dbl, "Current Description"=→"Current Description":string, "error out"=w1113:errorcluster, "JYMONOLib.IJYMonoReqd"=w1114:refnum<k7>)  [unwired: 6 in, 4 out]
          }
          frame #1 {
            n607 = call "JYGetCurrentWL.vi"("error in (no error)"=w1120, "JYMONOLib.IJYMonoReqd"=w1121) -> ("error out"=w1118:errorcluster, "Units"=→"Units":string, "Current WL"=→"Current WL":dbl, "JYMONOLib.IJYMonoReqd 2"=w1119:refnum<k7>)  [unwired: 6 in]
          }
          frame #2 {
            w1129 = u16 1 items=["Entrance", "Exit"] ("Mirror Number")
            w1130 = u16 0 items=["Entrance", "Exit"] ("Mirror Number")
            n608 = call "JYGetMirrorPos.vi"("error in (no error)"=w1131, "Mirror"=w1130, "Refnum In"=w1132) -> ("error out"=w1127:errorcluster, "Current Mirror Position"=→"Entrance Mirror\nPosition":i32, "Refnum Out"=w1128:refnum<k7>)  [unwired: 1 in]
            n609 = call "JYGetMirrorPos.vi"("error in (no error)"=w1127, "Mirror"=w1129, "Refnum In"=w1128) -> ("error out"=w1123:errorcluster, "Current Mirror Position"=→"Exit Mirror\nPosition":i32, "Refnum Out"=w1124:refnum<k7>)  [unwired: 1 in]
          }
          frame #3 {
            w1137 = u16 0 items=["Front Entrance", "Side Entrance", "Front Exit", "Side Exit", "First Intermediate", "Second Intermediate"] ("Slit")
            n610 = call "JYGetSlits.vi"("MonoRefNum IN"=w1135, "Slit"=w1137, "error in (no error)"=w1134) -> ("Units"=→"Units 2":string, "Slit Width"=→"Front Entrance":dbl, "error out"=→"error out":errorcluster)  [unwired: 13 in, 1 out]
          }
          frame #4 {
            n611 = case shown="假" "Move To\nTarget Positions" {
              tunnel: w1140 -> [_ w1141]
              frame False {
              }
              frame True {
                n612 = stacked-sequence {
                  seq-local: [w1143 _ _ _] -> [_ w1149 _ _]
                  seq-local: [_ w1147 _ _] -> [_ _ w1164 _]
                  seq-local: [_ _ w1151 _] -> [_ _ _ w1170]
                  seq-local: [_ _ _ w1167] -> [_ _ _ _]
                  tunnel: w1141 -> [w1145 w1148 w1162 w1171]
                  frame #0 {
                    n613 = property on="Target Grating" class="CmbBox"() -> ("Value"=w1142:string)  [unwired: 2 in, 2 out]
                    n614 = local read "error out"() -> (w1144:errorcluster)
                    n615 = Decimal String To Number(string=w1142) -> (number=w1146:i32)  [unwired: 2 in, 1 out]
                    n616 = call "JYTurret.vi"("error in (no error)"=w1144, "Grating Index"=w1146, "JYMONOLib.IJYMonoReqd"=w1145) -> ("error out"=w1143:errorcluster)  [unwired: 2 out]
                  }
                  frame #1 {
                    # "Move Grating to Target Position"
                    n617 = call "JYMoveToWavelength.vi"("error in (no error)"=w1149, "Target WL"="Target WL", "RefNum In"=w1148) -> ("error out"=w1147:errorcluster)  [unwired: 1 in, 2 out]
                  }
                  frame #2 {
                    w1157 = u16 1 items=["Entrance", "Exit"] ("Mirror Number")
                    w1156 = u16 0 items=["Entrance", "Exit"] ("Mirror Number")
                    w1163 = u16 1 items=["Entrance", "Exit", "Front", "Side"] ("Mirror Number")
                    w1166 = u16 0 items=["Entrance", "Exit", "Front", "Side"] ("Mirror Number")
                    # "Move Mirrors"
                    n618 = call "JYMirrorMove.vi"("error in (no error)"=w1164, "Mirror Position"="Entrance Mirror", "Mirror Number"=w1166, "RefNum In"=w1162) -> ("error out"=w1161:errorcluster)  [unwired: 6 in, 1 out]
                    n619 = call "JYMirrorMove.vi"("error in (no error)"=w1161, "Mirror Position"="Exit Mirror", "Mirror Number"=w1163, "RefNum In"=w1162) -> ("error out"=w1154:errorcluster, "MonoRefNum Out"=w1155:refnum<k7>)  [unwired: 6 in]
                    n620 = call "JYGetMirrorPos.vi"("error in (no error)"=w1154, "Mirror"=w1156, "Refnum In"=w1155) -> ("error out"=w1159:errorcluster, "Current Mirror Position"=w1153:i32, "Refnum Out"=w1158:refnum<k7>)  [unwired: 1 in]
                    n621 = local write "Entrance Mirror\nPosition"(w1153) -> ()
                    n622 = call "JYGetMirrorPos.vi"("error in (no error)"=w1159, "Mirror"=w1157, "Refnum In"=w1158) -> ("error out"=w1151:errorcluster, "Current Mirror Position"=w1152:i32)  [unwired: 1 in, 1 out]
                    n623 = local write "Exit Mirror\nPosition"(w1152) -> ()
                  }
                  frame #3 {
                    w1169 = u16 0 items=["Front Entrance", "Side Entrance", "Front Exit", "Side Exit", "First Intermediate", "Second Intermediate"] ("Slit")
                    # "Set New Slit Positions"
                    n624 = call "JYSlits.vi"("JYMONOLib.IJYMonoReqd"=w1171, "Slit"=w1169, "error in (no error)"=w1170, "Slit Width"="Target\nFront Entrance") -> ("error out"=w1167:errorcluster)  [unwired: 1 in, 1 out]
                  }
                }
              }
            }
          }
        }
        n625 = local read "Close"() -> (w1109:bool)
      }
    }
  }
  n626 = flat-sequence {
    frame #0 {
      n627 = call <vilib>:"Create Report.vi"("window state (normal)"=T3."no change", "report type"=Report_Type."Excel", "template (empty)"=path "D:/desktop/train/TEST1/Save/516中心波长.xlsx") -> ("report out"=w1178:refnum<class "NI_report.lvclass">, "error out"=w1177:errorcluster)  [unwired: 11 in]
      n628 = call-poly <vilib>:"Excel Get Data.vi"("report in"=w1178, "data type"=string[][] [], "error in (no error)"=w1177) -> ("report out"=w1173:refnum<class "NI_report.lvclass">, "data"=w1181:string[][], "error out"=w1172:errorcluster)  [unwired: 10 in]
      n629 = call-dynamic "Dispose Report.vi"("report in"=w1173, "error in (no error)"=w1172) -> ()  [unwired: 13 in, 1 out]
      n630 = Index Array(array=w1181, index (col)=0 ("禁用的索引 (列)")) -> (element=w1183:string[])  [unwired: 1 in]
      n631 = Fract/Exp String To Number(string=w1183) -> (number=→"波长范围":dbl[])  [unwired: 3 in, 1 out]
    }
  }
